vi "CaseSelect.vi"(10 "SelList[]":refnum<vi>[](array[refnum]), 11 "Active VI Ref":refnum<vi>) -> ()   [LabVIEW 2013]
uses:
  Controls/btn-back-36x36.ctl
  Controls/btn-forward-36x36.ctl
  Controls/btn-clear-history-36x36.ctl
  Controls/btn-refresh-36x36.ctl
  <vilib>/Utility/miscctls.llb/LVRectTypeDef.ctl
  StructureTypes.ctl
  JKI State Machine API/source/JKI SM/JKI SM.lvclass
  <vilib>/Utility/traverseref.llb/TRef TravTarget.ctl
  <userlib>/_OpenG.lib/comparison/comparison.llb/String Changed__ogtk.vi
  <userlib>/_OpenG.lib/comparison/comparison.llb/1D String Array Changed__ogtk.vi
  <userlib>/_OpenG.lib/file/file.llb/Build Path - File Names Array - path__ogtk.vi
  <vilib>/regexp/Match Regular Expression.xnode
  <userlib>/_OpenG.lib/string/string.llb/Trim Whitespace (String Array)__ogtk.vi
panel:
  in  "Refresh":T1
  in  "Clear History":T2
  in  "Forward":T3
  in  "Back":T4
  in  "Search Icon":bool
  in  "Clear Search":bool
  in  "Search":string
  in  "Add macro":bool
  in  "Cases":string(tree)
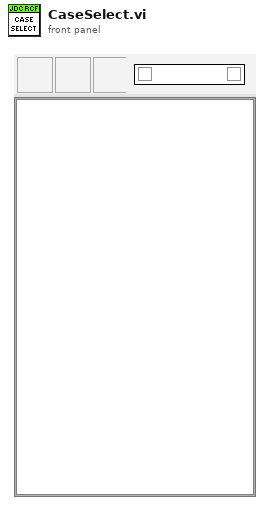
[diagram p1: front panel]
types:
  T1 = typedef "btn-refresh-36x36.ctl" = bool
  T2 = typedef "btn-clear-history-36x36.ctl" = bool
  T3 = typedef "btn-forward-36x36.ctl" = bool
  T4 = typedef "btn-back-36x36.ctl" = bool
  T5 = enum32{"Invalid", "Standard", "Closed", "Hidden", "Minimized", "Maximized"}
  T6 = enum32{"invalid app kind", "Development System", "Run Time System", "Student Edition", "Embedded LabVIEW", "Evaluation", "Custom"}
  T7 = typedef "StructureTypes.ctl" = enum16{"CaseStructure", "EventStructure"}
  T8 = typedef "TRef TravTarget.ctl" = enum16{"FP", "BD", "Other"}
  T9 = typedef "LVPoint32TypeDef.ctl" = cluster{"Horizontal":i32, "Vertical":i32}
  T10 = typedef "LVNodeAndColumnTypeDef.ctl" = cluster{"Node":string, "Column":i32}
  T11 = typedef "LVRectTypeDef.ctl" = cluster{"Left":i16, "Top":i16, "Right":i16, "Bottom":i16}
  T12 = cluster{"Core":cluster{"Current VI Reference":refnum<vi>, "Close Panel on Exit?":bool}, "Indent?":bool, "InBounds":bool, "Activating":bool, "FrameNames":string[], "tag":string, "Top Row Tag":string, "TreeSectHdrs":string, "SectHdr":string, "CaseStrVIName":string, "TempString":string, "DisplayedItems":i32, "SelectedCase":u32, "Display:Primary Workspace":T11, "Cases":refnum<vi>, "StructRef":refnum<vi>, "CaseStrVI Ref":refnum<vi>, "Ctrl?":bool, "NavHist":refnum<vi>[], "NavIndex":i32, "Structure Type":T7, "Undo Transaction":bool, "Top Row Index":i32}
  T13 = cluster{"Current VI Reference":refnum<vi>, "Close Panel on Exit?":bool}
  T14 = enum8{"Enabled", "Disabled", "Disabled and Grayed Out"}
  T15 = cluster{"StringConstant":refnum<vi>, "Structure":string, "Frame Name":string}[]
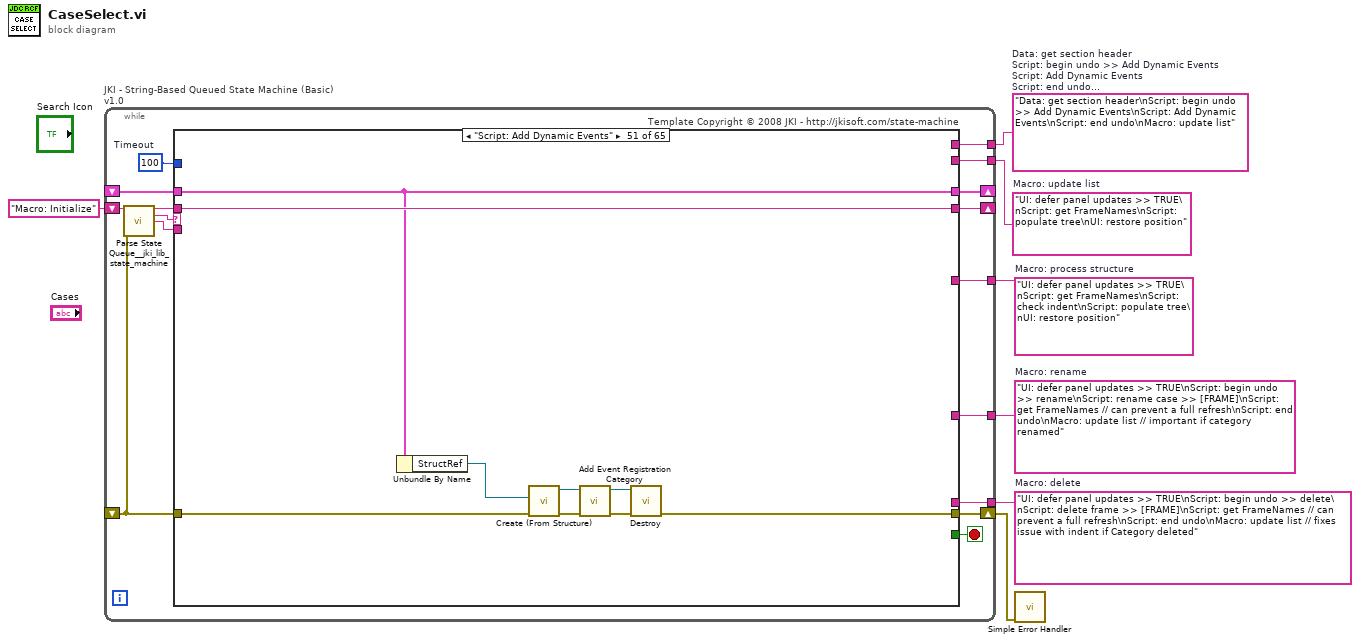
[diagram p0: block diagram]
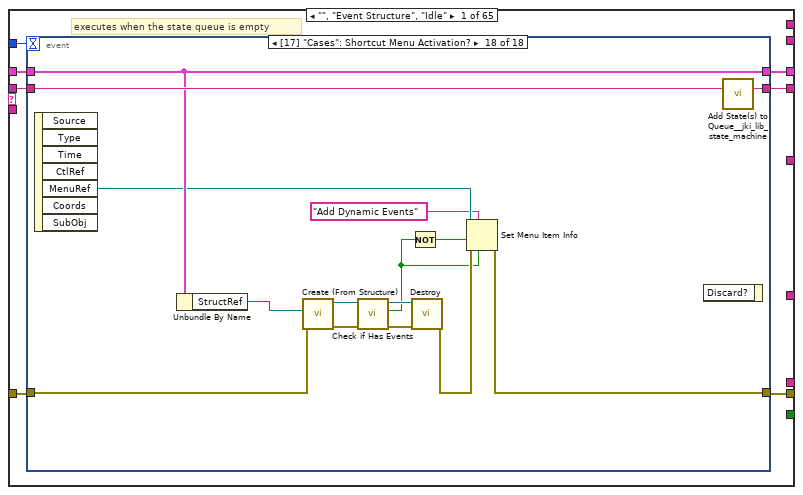
[diagram p2: hidden frame]
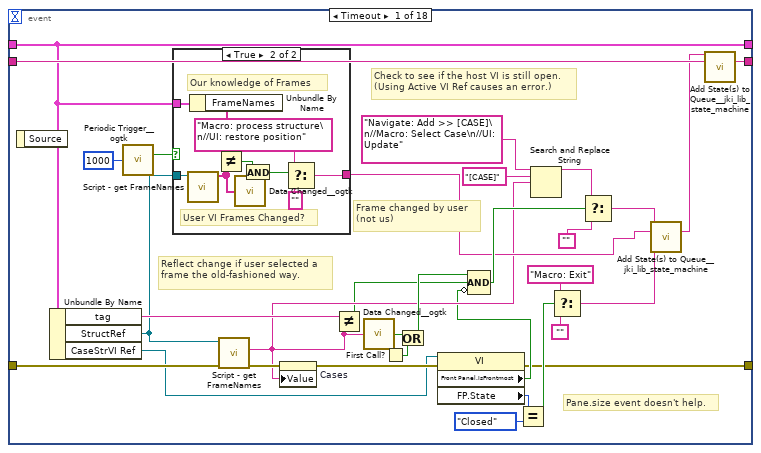
[diagram p3: hidden frame]
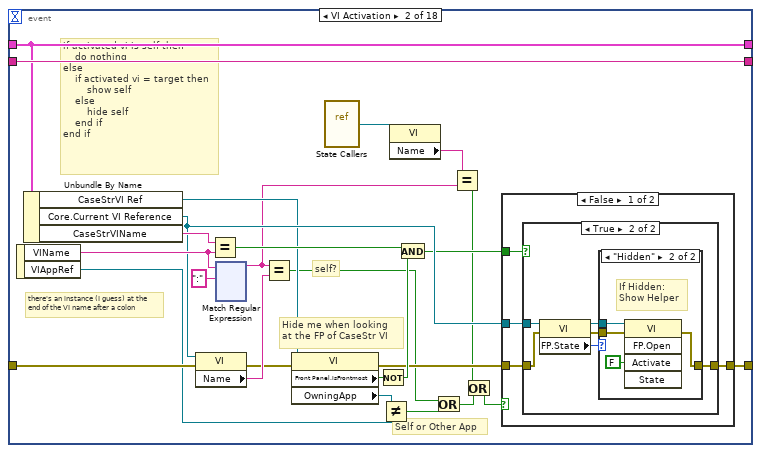
[diagram p5: hidden frame]
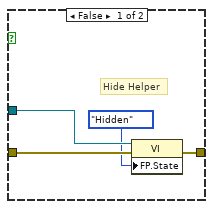
[diagram p6: hidden frame]
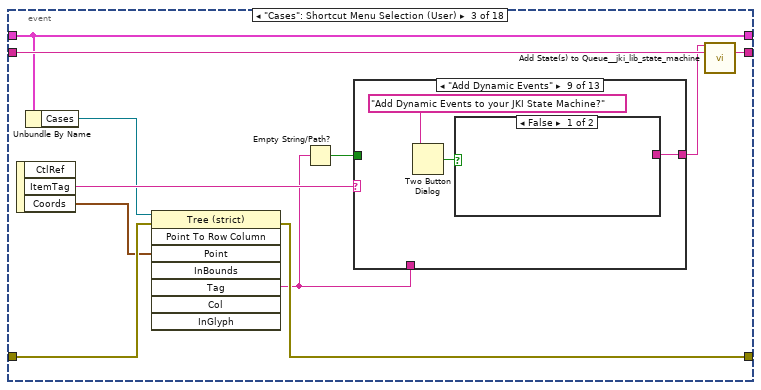
[diagram p9: hidden frame]
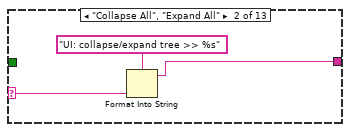
[diagram p11: hidden frame]
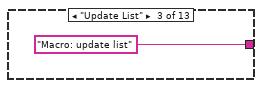
[diagram p12: hidden frame]
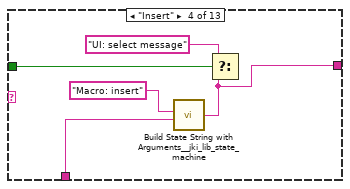
[diagram p13: hidden frame]
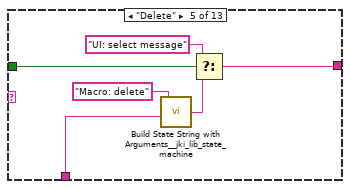
[diagram p14: hidden frame]
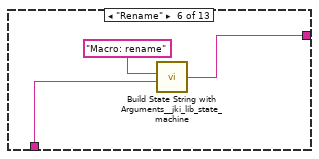
[diagram p15: hidden frame]
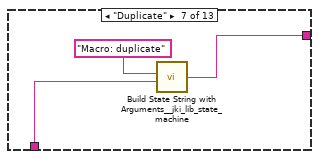
[diagram p16: hidden frame]
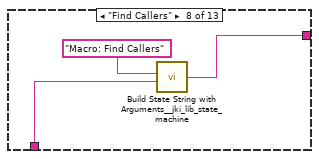
[diagram p17: hidden frame]
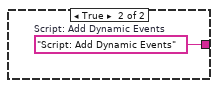
[diagram p18: hidden frame]
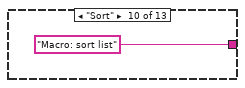
[diagram p19: hidden frame]
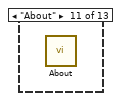
[diagram p20: hidden frame]
diagram:
  w1 = "Data: get section header\nScript: begin undo >> Add Dynamic Events\nScript: Add Dynamic Events\nScript: end undo\nMacro: update list"  # Data: get section header Script: begin undo >> Add Dynamic Events Script: Add Dynamic Events Script: end undo Macro: update list
  w2 = "UI: defer panel updates >> TRUE\nScript: get FrameNames\nScript: populate tree\nUI: restore position"  # Macro: update list
  w4 = "UI: defer panel updates >> TRUE\nScript: begin undo >> delete\nScript: delete frame >> [FRAME]\nScript: get FrameNames // can prevent a full refresh\nScript: end undo\nMacro: update list // fixes issue with indent if Category deleted"  # Macro: delete
  w5 = "UI: defer panel updates >> TRUE\nScript: begin undo >> rename\nScript: rename case >> [FRAME]\nScript: get FrameNames // can prevent a full refresh\nScript: end undo\nMacro: update list // important if category renamed"  # Macro: rename
  w6 = "UI: defer panel updates >> TRUE\nScript: get FrameNames\nScript: check indent\nScript: populate tree\nUI: restore position"  # Macro: process structure
  n1 = while "JKI - String-Based Queued State Machine (Basic) v1.0" {
    shift-right: [w16] -> _
    shift-left: _ -> [w15]
    shift-right: [w19] -> w3
    shift-left: _ -> [w13]
    shift-right: [w18] -> _
    shift-left: "Macro: Initialize" -> [w20]
    tunnel: w6 -> [w12]
    tunnel: w5 -> [w11]
    tunnel: w4 -> [w10]
    tunnel: w2 -> [w9]
    tunnel: w1 -> [w8]
    stop <- w17 stop-if-true
    w14 = 100  # Timeout
    # "Template Copyright © 2008 JKI - http://jkisoft.com/state-machine"
    n2 = call <vilib>:"Parse State Queue__jki_lib_state_machine.vi"("State Queue"=w20, "Error In (no error)"=w13) -> ("Remaining States"=w22:string, "Current State"=w23:string, "Arguments"=w21:string)  [unwired: 1 in, 10 out]
    n3 = case shown="\"Script: Add Dynamic Events\"" w23 {
      selector: w23 -> [_ _ w509 _ _ _ _ _ _ _ _ _ _ _ _ _ _ _ _ _ _ _ _ _ _ _ _ _ _ _ _ _ _ _ _ _ _ _ _ _ _ _ _ _ _ _ _ _ _ _ _ _ _ _ _ _ _ _ _ _ _ _ _ _ _]
      tunnel: w22 -> [w30 w505 w508 w518 w537 _ w560 w564 w574 w618 w635 w644 w647 w655 w672 w674 w716 w726 w744 w759 w787 w810 w812 w819 w822 w830 w840 w861 w864 w870 w874 w885 w893 w898 w907 w911 w916 w926 w933 w934 w947 w964 w965 w975 w998 w1015 w1017 w1041 w1081 w1099 w1108 w1117 w1184 w1244 w1316 w1393 w1430 w1456 w1489 w1513 w1521 w1527 w1535 w1550 w1600]
      tunnel: w21 -> [_ _ _ _ _ _ _ _ _ _ _ _ _ _ _ w673 _ w729 _ w761 _ _ _ _ _ w825 w836 w857 _ _ _ w878 w890 _ w904 _ _ w923 _ _ w937 _ _ w972 _ _ _ _ _ _ _ w1110 w1176 w1234 w1307 w1387 w1423 _ w1493 _ _ _ _ _ _]
      tunnel: w15 -> [w28 w506 w511 w521 w538 w548 w563 w565 _ w617 w633 w645 w648 w656 w670 w676 w715 w731 w748 w762 w786 w809 w813 w816 w823 w831 w841 w853 w865 w868 w876 w879 w894 w899 w908 w913 w918 w928 w930 w935 w945 w961 w966 w973 w997 w1013 w1025 w1040 w1080 w1098 w1107 w1119 w1188 w1236 w1319 w1396 w1431 w1468 w1495 w1514 w1520 w1526 w1534 w1560 w1599]
      tunnel: [w27 w507 w513 w527 w539 w550 w562 w566 w575 w619 w634 w642 w649 w654 w671 w677 w713 w732 w749 w764 w785 w811 w814 w817 w824 w832 w834 w856 w866 w871 w875 w881 w888 w896 w902 w912 w917 w927 w931 w936 w942 w957 w967 w974 w991 w1008 w1018 w1042 w1079 w1097 w1100 w1113 w1187 w1245 w1317 w1394 w1420 w1460 w1479 w1512 w1517 w1523 w1531 w1553 w1594] -> w19
      tunnel: w13 -> [w26 w507 w512 w527 w539 w554 w562 w566 w589 w619 w634 w643 w649 w654 w671 w678 w714 w733 w750 w763 w788 w811 w814 w817 w824 w832 w835 w844 w866 w871 w875 w882 w889 w896 w903 w912 w917 w927 w931 w936 w943 w958 w967 w971 w993 w1016 w1019 w1043 w1073 w1096 w1101 w1120 w1189 w1242 w1312 w1389 w1421 w1466 w1478 w1512 w1519 w1525 w1533 w1559 w1596]
      tunnel: [w29 w505 w508 w518 w537 w546 w560 w564 w574 w618 w635 w644 w647 w655 w672 w674 w716 w725 w743 w758 w787 w810 w812 w818 w821 w829 w839 w860 w863 w869 w873 w884 w892 w897 w906 w910 w915 w925 w932 w934 w947 w964 w965 w975 w998 w1014 w1017 w1041 w1081 w1099 w1108 w1116 w1183 w1244 w1315 w1392 w1429 w1455 w1488 w1513 w1521 w1527 w1535 w1549 w1600] -> w18
      tunnel: [_ _ _ _ _ _ TRUE _ _ _ _ _ _ _ _ _ _ _ _ _ _ _ _ _ _ _ _ _ _ _ _ _ _ _ _ _ _ _ _ _ _ _ _ _ _ _ _ _ _ _ _ _ _ _ _ _ _ _ _ _ _ _ _ _ _] -> w17
      tunnel: [w25 w506 w511 w528 w538 w548 w563 w565 w599 w616 w629 w645 w648 w656 w670 w676 w715 w731 w745 w762 w786 w809 w813 w816 w823 w831 w841 w853 w865 w868 w876 w879 w894 w899 w908 w913 w918 w928 w930 w935 w946 w960 w966 w969 w995 w1011 w1024 w1039 w1076 w1098 w1107 w1119 w1188 w1235 w1319 w1396 w1431 w1454 w1483 w1514 w1516 w1526 w1530 w1560 w1599] -> w16
      tunnel: w14 -> [w24 _ _ _ _ _ _ _ _ _ _ _ _ _ _ _ _ _ _ _ _ _ _ _ _ _ _ _ _ _ _ _ _ _ _ _ _ _ _ _ _ _ _ _ _ _ _ _ _ _ _ _ _ _ _ _ _ _ _ _ _ _ _ _ _]
      tunnel: w12 -> [_ _ _ _ _ _ _ _ _ _ _ _ _ _ _ _ _ _ _ _ _ _ _ _ w820 _ _ _ _ _ _ _ _ _ _ _ _ _ _ _ _ _ _ _ _ _ _ _ _ _ _ _ _ _ _ _ _ _ _ _ _ _ _ _ _]
      tunnel: w11 -> [_ _ _ _ _ _ _ _ _ _ _ _ _ _ _ _ _ _ _ _ _ _ _ _ _ _ _ _ _ _ _ w877 _ _ _ _ _ _ _ _ _ _ _ _ _ _ _ _ _ _ _ _ _ _ _ _ _ _ _ _ _ _ _ _ _]
      tunnel: w10 -> [_ _ _ _ _ _ _ _ _ _ _ _ _ _ _ _ _ _ _ _ _ _ _ _ _ _ w833 _ _ _ _ _ _ _ _ _ _ _ _ _ _ _ _ _ _ _ _ _ _ _ _ _ _ _ _ _ _ _ _ _ _ _ _ _ _]
      tunnel: w9 -> [_ _ _ _ _ _ _ _ _ _ _ _ _ _ _ _ _ _ _ _ _ _ _ _ _ _ _ _ w862 _ _ _ _ _ _ _ _ _ _ _ _ _ _ _ _ _ _ _ _ _ _ _ _ _ _ _ _ _ _ _ _ _ _ _ _]
      tunnel: w8 -> [_ _ _ _ _ _ _ _ _ _ _ _ _ _ _ _ _ _ _ _ _ _ _ _ _ _ _ _ _ _ _ _ _ w895 _ _ _ _ _ _ _ _ _ _ _ _ _ _ _ _ _ _ _ _ _ _ _ _ _ _ _ _ _ _ _]
      frame "", "Event Structure", "Idle" {
        # "executes when the state queue is empty"
        n4 = event shown="[17] \"Cases\": Shortcut Menu Activation?" {
          selector: _ -> [_ _ _ _ _ _ _ _ _ _ _ _ _ _ _ _ _ _]
          dyn-events: _ -> [_ _ _ _ _ _ _ _ _ _ _ _ _ _ _ _ _ _]
          timeout: w24 -> [_ _ _ _ _ _ _ _ _ _ _ _ _ _ _ _ _ _]
          tunnel: w30 -> [w62 w98 w238 w294 w323 w332 w338 w366 w401 w403 w411 w419 w434 w453 w456 w463 w489 w504]
          tunnel: [w61 w98 w237 w293 w322 w332 w337 w365 w401 w402 w410 w418 w433 w452 w457 w463 w488 w503] -> w29
          tunnel: w28 -> [w31 w96 w235 w296 w324 w331 w335 w367 w399 w406 w414 w422 w447 w450 w458 w464 w486 w497]
          tunnel: [w32 w94 w231 w283 w320 w327 w339 w368 w400 w405 w413 w421 w435 w454 w459 w460 w487 w492] -> w27
          tunnel: w26 -> [w60 w86 w240 w298 w320 w328 w340 w368 w400 w405 w413 w421 w426 w454 w459 w461 w487 w496]
          tunnel: [w31 w96 w235 w287 w321 w326 w335 w363 w399 w406 w414 w422 w448 w450 w458 w462 w486 w497] -> w25
          event Timeout {
            # "Frame changed by user\n(not us)"
            # "Reflect change if user selected a frame the old-fashioned way."
            # "Pane.size event doesn't help."
            # "Check to see if the host VI is still open.\n(Using Active VI Ref causes an error.)"
            n5 = event-data() -> ()  [unwired: 2 out]
            n6 = Unbundle By Name(w31) -> ("tag"=w53:string, "StructRef"=w39:refnum<vi>, "CaseStrVI Ref"=w40:refnum<vi>)
            n7 = call <userlib>:"Periodic Trigger__ogtk.vi"("time (ms)"=u32 1000) -> ("Triggered"=w42:bool)  [unwired: 12 in, 2 out]
            n8 = case shown="True" w42 {
              tunnel: w39 -> [_ w72]
              tunnel: [_ w69] -> w41
              tunnel: w31 -> [_ w68]
              frame False {
              }
              frame True {
                # "Our knowledge of Frames"
                # "User VI Frames Changed?"
                n9 = call "Script - get FrameNames.vi"("StructRef"=w72) -> ("Frame Names"=w67:string[])  [unwired: 5 in, 5 out]
                n10 = Unbundle By Name(w68) -> ("FrameNames"=w66:string[])
                n11 = Not Equal?(x=w66, y=w67) -> (x != y?=w64:bool)
                n12 = call-poly <userlib>:"Data Changed__ogtk.vi"("1D String Array"=w67) -> ("Changed"=w63:bool)
                n13 = And(x=w64, y=w63) -> (x .and. y?=w65:bool)
                n14 = Select(t="Macro: process structure\n//UI: restore position", s=w65, f="") -> (s? t:f=w69:string)
              }
            }
            n15 = call "Script - get FrameNames.vi"("error in"=w60, "StructRef"=w39) -> ("error out"=w38:errorcluster, "Visible Frame Name"=w37:string)  [unwired: 4 in, 4 out]
            n16 = property on="Cases" class="Tree (strict)"(error in=w38, "Value"=w37) -> (error out=w54:errorcluster)  [unwired: 1 in, 1 out]
            n17 = Not Equal?(x=w53, y=w37) -> (x != y?=w33:bool)
            n18 = call-poly <userlib>:"Data Changed__ogtk.vi"("String"=w37) -> ("Changed"=w45:bool)
            n19 = First Call?() -> (First Call?: T/F=w46:bool)
            n20 = Or(x=w45, y=w46) -> (x .or. y?=w44:bool)
            n21 = property class="VI"(reference=w40, error in=w54) -> (error out=w32:errorcluster, "Front Panel.IsFrontmost"=w34:bool, "FP.State"=w59:T5)  [unwired: 1 out]
            n22 = Compound Arithmetic op=AND(w44, w33, invert w34) -> (w49:bool)
            n23 = Equal?(x=w59, y=T5."Closed" ("Front Panel Window:State")) -> (x = y?=w57:bool)
            n24 = Search and Replace String(input string="Navigate: Add >> [CASE]\n//Macro: Select Case\n//UI: Update" ("State(s) in Front (\"\")"), search string="[CASE]", replace string=w37) -> (result string=w36:string)  [unwired: 5 in, 3 out]
            n25 = Select(t="Macro: Exit", s=w57, f="") -> (s? t:f=w48:string)
            n26 = Select(t=w36, s=w49, f="") -> (s? t:f=w35:string)
            n27 = call <vilib>:"Add State(s) to Queue__jki_lib_state_machine.vi"("State(s) in Front (\"\")"=w35, "State(s) in (\"\")"=w41, "State(s) at Back (\"\")"=w48) -> ("States Out"=w47:string)  [unwired: 12 out]
            n28 = call <vilib>:"Add State(s) to Queue__jki_lib_state_machine.vi"("State(s) in Front (\"\")"=w47, "State(s) in (\"\")"=w62) -> ("States Out"=w61:string)  [unwired: 1 in, 12 out]
          }
          event VI Activation {
            # "Self or Other App"
            # "self?"
            # "Hide me when looking\nat the FP of CaseStr VI"
            # "there's an instance (I guess) at the\nend of the VI name after a colon"
            # "if activated vi is self then\n    do nothing\nelse\n    if activated vi = target then\n        show self\n    else\n        hide self\n    end if\nend if"
            n29 = event-data() -> ("VIName"=w91:string, "VIAppRef"=w81:refnum<vi>)  [unwired: 1 out]
            n30 = Unbundle By Name(w96) -> ("CaseStrVI Ref"=w84:refnum<vi>, "Core.Current VI Reference"=w90:refnum<vi>, "CaseStrVIName"=w97:string)
            n31 = property class="VI"(reference=w90, error in=w86) -> (error out=w85:errorcluster, "Name"=w92:string)  [unwired: 1 out]
            n32 = Equal?(x=w97, y=w91) -> (x = y?=w95:bool)
            n33 = xnode "Match Regular Expression"("input string"=w91, "regular expression"=":") -> ("before match"=w76:string)  [unwired: 3 in, 5 out]
            n34 = Equal?(x=w76, y=w92) -> (x = y?=w79:bool)
            n35 = property class="VI"(reference=w84, error in=w85) -> (error out=w87:errorcluster, "Front Panel.IsFrontmost"=w89:bool, "OwningApp"=w82:refnum<vi>)  [unwired: 1 out]
            n36 = vi-ref "State Callers.vi"() -> (w78:refnum<vi>)
            n37 = Not(x=w89) -> (.not. x?=w88:bool)
            n38 = Not Equal?(x=w82, y=w81) -> (x != y?=w80:bool)
            n39 = property class="VI"(reference=w78) -> ("Name"=w77:string)  [unwired: 1 in, 2 out]
            n40 = And(x=w95, y=w88) -> (x .and. y?=w83:bool)
            n41 = Or(x=w79, y=w80) -> (x .or. y?=w74:bool)
            n42 = Equal?(x=w77, y=w76) -> (x = y?=w75:bool)
            n43 = Or(x=w75, y=w74) -> (x .or. y?=w73:bool)
            n44 = case shown="False" w73 {
              tunnel: w87 -> [w102 w118]
              tunnel: [w100 w118] -> w94
              tunnel: w90 -> [w101 _]
              tunnel: w83 -> [w99 _]
              frame False {
                n45 = case shown="True" w99 {
                  tunnel: w102 -> [w106 w111]
                  tunnel: w101 -> [w105 w112]
                  tunnel: [w104 w109] -> w100
                  frame False {
                    # "Hide Helper"
                    n46 = property class="VI"(reference=w105, error in=w106, "FP.State"=T5."Hidden" ("Front Panel Window:State")) -> (error out=w104:errorcluster)  [unwired: 1 out]
                  }
                  frame True {
                    n47 = property class="VI"(reference=w112, error in=w111) -> (reference out=w108:refnum<vi>, error out=w107:errorcluster, "FP.State"=w110:T5)
                    n48 = case shown="\"Hidden\"" w110 {
                      tunnel: [w113 w117] -> w109
                      tunnel: w108 -> [_ w116]
                      tunnel: w107 -> [w113 w115]
                      frame Default {
                      }
                      frame "Hidden" {
                        # "If Hidden:\nShow Helper"
                        n49 = invoke class="VI" method="FP.Open"(reference=w116, error in=w115, "Activate"=FALSE ("Activate?")) -> (error out=w117:errorcluster)  [unwired: 2 in, 4 out]
                      }
                    }
                  }
                }
              }
              frame True {
              }
            }
          }
          event "Cases": Shortcut Menu Selection (User) {
            n50 = event-data() -> ("ItemTag"=w239:string, "Coords"=w232:T9)  [unwired: 2 out]
            n51 = Unbundle By Name(w235) -> ("Cases"=w234:refnum<vi>)
            n52 = invoke class="Tree (strict)" method="Point To Row Column"(reference=w234, error in=w240, "Point"=w232) -> (error out=w231:errorcluster, "Tag"=w230:string)  [unwired: 5 in, 6 out]
            n53 = Empty String/Path?(string/path=w230) -> (empty?=w233:bool)
            n54 = case shown="\"Add Dynamic Events\"" w239 {
              selector: w239 -> [_ w242 _ _ _ _ _ _ _ _ _ _ _]
              tunnel: [_ w241 "Macro: update list" w245 w253 w256 w259 w262 w267 "Macro: sort list" _ w270 _] -> w236
              tunnel: w233 -> [_ _ _ w249 w255 _ _ _ _ _ _ _ _]
              tunnel: w230 -> [_ _ _ w246 w251 w258 w261 w264 _ _ _ _ w276]
              frame Default {
              }
              frame "Collapse All", "Expand All" {
                n55 = Format Into String(format string="UI: collapse/expand tree >> %s", w242) -> (resulting string=w241:string)  [unwired: 2 in, 1 out]
              }
              frame "Update List" {
              }
              frame "Insert" {
                n56 = call <vilib>:"Build State String with Arguments__jki_lib_state_machine.vi"("Arguments (\"\")"=w246, "State"="Macro: insert") -> ("State with Arguments"=w245:string)  [unwired: 4 in]
                n57 = Select(t="UI: select message", s=w249, f=w245) -> ()  [unwired: 1 out]
              }
              frame "Delete" {
                n58 = call <vilib>:"Build State String with Arguments__jki_lib_state_machine.vi"("Arguments (\"\")"=w251, "State"="Macro: delete") -> ("State with Arguments"=w250:string)  [unwired: 4 in]
                n59 = Select(t="UI: select message", s=w255, f=w250) -> (s? t:f=w253:string)
              }
              frame "Rename" {
                n60 = call <vilib>:"Build State String with Arguments__jki_lib_state_machine.vi"("Arguments (\"\")"=w258, "State"="Macro: rename") -> ("State with Arguments"=w256:string)  [unwired: 4 in]
              }
              frame "Duplicate" {
                n61 = call <vilib>:"Build State String with Arguments__jki_lib_state_machine.vi"("Arguments (\"\")"=w261, "State"="Macro: duplicate") -> ("State with Arguments"=w259:string)  [unwired: 4 in]
              }
              frame "Find Callers" {
                n62 = call <vilib>:"Build State String with Arguments__jki_lib_state_machine.vi"("Arguments (\"\")"=w264, "State"="Macro: Find Callers") -> ("State with Arguments"=w262:string)  [unwired: 4 in]
              }
              frame "Add Dynamic Events" {
                n63 = Two Button Dialog(message="Add Dynamic Events to your JKI State Machine?" ("format string")) -> (T button?=w266:bool)  [unwired: 2 in]
                n64 = case shown="False" w266 {
                  tunnel: [_ w268] -> w267
                  frame False {
                  }
                  frame True {
                    w268 = "Script: Add Dynamic Events"  # Script: Add Dynamic Events
                  }
                }
              }
              frame "Sort" {
              }
              frame "About" {
                n65 = call "About.vi"() -> ()  [unwired: 1 out]
              }
              frame "highlight" {
                w270 = "Script: highlight"  # Script: highlight
              }
              frame "Copy State Name to Clipboard" {
                # "Don't trim quotes"
                n66 = call <vilib>:"Trim Whitespace.vi"("string"=w276) -> ("trimmed string"=w273:string)  [unwired: 1 in]
                n67 = Equal?(x=string[] ["\"\", \"Idle\"", " \"\", \"Event Structure\", \"Idle\" "], y=w273) -> (x = y?=w275:bool[])
                n68 = call "Remove Quotes from String if Present.vi"("String"=w273) -> ("String with Quotes Removed"=w272:string)  [unwired: 10 in]
                n69 = Or Array Elements(Boolean array=w275) -> (logical OR=w274:bool)
                n70 = Select(t=w273, s=w274, f=w272) -> (s? t:f=w271:string)
                n71 = invoke class="App" method="Clipboard.Write"("Param 0"=w271) -> ()  [unwired: 3 in, 4 out]
              }
            }
            n72 = call <vilib>:"Add State(s) to Queue__jki_lib_state_machine.vi"("State(s) in Front (\"\")"=w236, "State(s) in (\"\")"=w238) -> ("States Out"=w237:string)  [unwired: 1 in, 12 out]
          }
          event "Cases": Drag Ended {
            n73 = event-data() -> ("CtlRef"=w297:refnum<vi>)  [unwired: 1 out]
            n74 = Unbundle By Name(w296) -> ("Ctrl?"=w280:bool, "FrameNames"=w291:string[], "StructRef"=w295:refnum<vi>, "CaseStrVI Ref"=w279:refnum<vi>)
            n75 = property class="Tree (strict)"(reference=w297, error in=w298) -> (error out=w292:errorcluster, "TopLeft"=w286:T10, "Value"=w282:string, "All Tags"=w284:string[])  [unwired: 1 out]
            n76 = Unbundle By Name(w286) -> ("Node"=w285:string)
            n77 = Array Size(array=w291) -> (size(s)=w289:i32)
            n78 = Array Size(array=w284) -> (size(s)=w290:i32)
            n79 = Bundle By Name(cluster=w296, "Top Row Tag"=w285, "tag"=w282) -> (w287:T12)
            n80 = Equal?(x=w289, y=w290) -> (x = y?=w288:bool)
            n81 = case shown="True" w288 {
              tunnel: w295 -> [_ w302]
              tunnel: w292 -> [w300 w309]
              tunnel: [w300 w305] -> w283
              tunnel: w291 -> [_ w311]
              tunnel: w284 -> [_ w310]
              tunnel: ["Macro: process drag-copy" ("message") "Macro: update list\nMacro: Select Case" ("message")] -> w278
              tunnel: w279 -> [_ w301]
              frame False {
                # "There are more tags in the tree than\nthere are frames in the Case Structure.\nA drag/copy operation just occurred."
              }
              frame True {
                n82 = for {
                  tunnel: w311 -> [w315]
                  tunnel: w310 -> [w314] mode=indexing
                  tunnel: [w313] -> w312 mode=indexing
                  n83 = Search 1D Array(1D array=w315, element=w314) -> (index of element=w313:i32)  [unwired: 1 out]
                }
                n84 = invoke class="VI" method="Transaction.Begin Undo"(reference=w301, error in=w309, "Name"="Drag") -> (reference out=w306:refnum<vi>, error out=w307:errorcluster)  [unwired: 1 in, 2 out]
                n85 = invoke class="MFStruct" method="RearrangeFramesByIdx"(reference=w302, error in=w307, "Index Array"=w312) -> (error out=w303:errorcluster)  [unwired: 1 in, 3 out]
                n86 = invoke class="VI" method="Transaction.End Undo"(reference=w306, error in=w303) -> (error out=w305:errorcluster)  [unwired: 1 in, 2 out]
              }
            }
            n87 = Select(t="Macro: drop state name", s=w280, f=w278) -> ()  [unwired: 1 out]
            n88 = call <vilib>:"Add State(s) to Queue__jki_lib_state_machine.vi"("State(s) in Front (\"\")"=w278, "State(s) in (\"\")"=w294) -> ("States Out"=w293:string)  [unwired: 1 in, 12 out]
          }
          event "Cases": Value Change {
            n89 = event-data() -> ("NewVal"=w317:string)  [unwired: 1 out]
            n90 = Bundle By Name(cluster=w324, "tag"=w317) -> (w321:T12)
            n91 = Search and Replace String(input string="Navigate: Add >> [CASE]\nMacro: Select Case\nUI: Update" ("State(s) in Front (\"\")"), search string="[CASE]", replace string=w317) -> (result string=w316:string)  [unwired: 5 in, 3 out]
            n92 = call <vilib>:"Add State(s) to Queue__jki_lib_state_machine.vi"("State(s) in Front (\"\")"=w316, "State(s) in (\"\")"=w323) -> ("States Out"=w322:string)  [unwired: 1 in, 12 out]
          }
          event "Cases": Mouse Down {
            # "This makes a mouse click work\nonly if the click was in bounds."
            n93 = event-data() -> ("CtlRef"=w330:refnum<vi>, "Coords"=w329:T9)  [unwired: 4 out]
            n94 = invoke class="Tree (strict)" method="Point To Row Column"(reference=w330, error in=w328, "Point"=w329) -> (error out=w327:errorcluster, "InBounds"=w325:bool)  [unwired: 5 in, 6 out]
            n95 = Bundle By Name(cluster=w331, "InBounds"=w325) -> (w326:T12)
          }
          event "Cases": Mouse Up {
            n96 = event-data() -> ("Mods.Double Click"=w333:bool, "PlatMods.Ctrl"=w334:bool, "CtlRef"=w342:refnum<vi>, "Coords"=w341:T9)  [unwired: 1 out]
            n97 = case shown="False" w333 {
              tunnel: w342 -> [w354 _]
              tunnel: w341 -> [w353 _]
              tunnel: w340 -> [w352 w356]
              tunnel: [w351 w356] -> w339
              tunnel: [w350 "//Macro: append string"] -> w336
              tunnel: w335 -> [w349 _]
              tunnel: w334 -> [w348 _]
              frame False {
                n98 = invoke class="Tree (strict)" method="Point To Row Column"(reference=w354, error in=w352, "Point"=w353) -> (error out=w351:errorcluster, "InBounds"=w346:bool)  [unwired: 5 in, 6 out]
                n99 = Unbundle By Name(w349) -> ("InBounds"=w347:bool)
                n100 = Compound Arithmetic op=AND(invert w348, w347, w346) -> (w345:bool)
                n101 = Select(t="//Macro: Select Case", s=w345, f="") -> (s? t:f=w350:string)
              }
              frame True {
              }
            }
            n102 = call <vilib>:"Add State(s) to Queue__jki_lib_state_machine.vi"("State(s) in Front (\"\")"=w336, "State(s) in (\"\")"=w338) -> ("States Out"=w337:string)  [unwired: 1 in, 12 out]
          }
          event Key Down? {
            n103 = event-data() -> ("PlatMods.Shift"=w359:bool, "PlatMods.Ctrl"=w361:bool, "ScanCode"=w360:i16)  [unwired: 1 out]
            n104 = Bundle By Name(cluster=w367, "Ctrl?"=w361) -> (w363:T12)
            n105 = Unbundle By Name(w363) -> ("tag"=w362:string, "CaseStrVI Ref"=w358:refnum<vi>)
            n106 = case shown="44" w360 {
              tunnel: [_ w370 w374 w378 w383 _] -> w364
              tunnel: w362 -> [_ w372 w376 w380 w384 w393]
              tunnel: w361 -> [_ _ _ _ w382 w392]
              tunnel: w359 -> [_ _ _ _ _ w391]
              tunnel: w358 -> [_ _ _ _ _ w390]
              tunnel: [_ TRUE TRUE TRUE w381 w389] -> w357
              frame 0, Default {
              }
              frame 60 {
                # "F2"
                n107 = call <vilib>:"Build State String with Arguments__jki_lib_state_machine.vi"("Arguments (\"\")"=w372, "State"="Macro: rename") -> ("State with Arguments"=w370:string)  [unwired: 4 in]
              }
              frame 82 {
                n108 = call <vilib>:"Build State String with Arguments__jki_lib_state_machine.vi"("Arguments (\"\")"=w376, "State"="Macro: insert") -> ("State with Arguments"=w374:string)  [unwired: 4 in]
              }
              frame 83 {
                # "Delete"
                n109 = call <vilib>:"Build State String with Arguments__jki_lib_state_machine.vi"("Arguments (\"\")"=w380, "State"="Macro: delete") -> ("State with Arguments"=w378:string)  [unwired: 4 in]
              }
              frame 33 {
                # "Ctrl+F"
                n110 = case shown="True" w382 {
                  tunnel: w384 -> [_ w388]
                  tunnel: [_ w386] -> w383
                  tunnel: [_ TRUE] -> w381
                  frame False {
                  }
                  frame True {
                    n111 = call <vilib>:"Build State String with Arguments__jki_lib_state_machine.vi"("Arguments (\"\")"=w388, "State"="Macro: Find Callers") -> ("State with Arguments"=w386:string)  [unwired: 4 in]
                  }
                }
              }
              frame 44 {
                # "Z"
                n112 = case shown="True" w392 {
                  tunnel: w393 -> [_ _]
                  tunnel: w391 -> [_ w396]
                  tunnel: w390 -> [_ w395]
                  tunnel: [_ TRUE] -> w389
                  frame False {
                  }
                  frame True {
                    # "Ctrl+Z"
                    n113 = case shown="True" w396 {
                      tunnel: w395 -> [w397 w398]
                      frame False {
                        n114 = invoke class="VI" method="Transaction.Undo"(reference=w397) -> ()  [unwired: 2 in, 3 out]
                      }
                      frame True {
                        n115 = invoke class="VI" method="Transaction.Redo"(reference=w398) -> ()  [unwired: 2 in, 3 out]
                      }
                    }
                  }
                }
              }
            }
            n116 = event-data("Discard?"=w357) -> ()  [unwired: 1 in, 1 out]
            n117 = call <vilib>:"Add State(s) to Queue__jki_lib_state_machine.vi"("State(s) in Front (\"\")"=w364, "State(s) in (\"\")"=w366) -> ("States Out"=w365:string)  [unwired: 1 in, 12 out]
          }
          event Mouse Leave {
            n118 = event-data() -> ()  [unwired: 5 out]
          }
          event Panel Resize {
            n119 = event-data() -> ()  [unwired: 4 out]
            n120 = call <vilib>:"Add State(s) to Queue__jki_lib_state_machine.vi"("State(s) in Front (\"\")"="UI: show/hide scroll bar", "State(s) in (\"\")"=w403) -> ("States Out"=w402:string)  [unwired: 1 in, 12 out]
          }
          event "Search": Value Change {
            n121 = event-data() -> ("NewVal"=w409:string)  [unwired: 6 out]
            n122 = Empty String/Path?(string/path=w409) -> (empty?=w407:bool)
            n123 = Not(x=w407) -> (.not. x?=w408:bool)
            n124 = property on="Search Icon" class="Bool (strict)"("Visible"=w407) -> ()  [unwired: 2 in, 2 out]
            n125 = property on="Clear Search" class="Bool (strict)"("Visible"=w408) -> ()  [unwired: 2 in, 2 out]
            n126 = call <vilib>:"Add State(s) to Queue__jki_lib_state_machine.vi"("State(s) in Front (\"\")"="Macro: process structure", "State(s) in (\"\")"=w411) -> ("States Out"=w410:string)  [unwired: 1 in, 12 out]
          }
          event "Clear Search": Value Change {
            n127 = event-data() -> ()  [unwired: 7 out]
            n128 = property on="Clear Search" class="Bool (strict)"("Visible"=FALSE) -> ()  [unwired: 2 in, 2 out]
            n129 = property on="Search Icon" class="Bool (strict)"("Visible"=TRUE) -> ()  [unwired: 2 in, 2 out]
            n130 = local write "Search"("" ("Search")) -> ()
            n131 = call <vilib>:"Add State(s) to Queue__jki_lib_state_machine.vi"("State(s) in Front (\"\")"="Macro: process structure", "State(s) in (\"\")"=w419) -> ("States Out"=w418:string)  [unwired: 1 in, 12 out]
          }
          event Value Change {
            n132 = event-data() -> ()  [unwired: 7 out]
            n133 = Unbundle By Name(w447) -> ("NavIndex"=w436:i32, "NavHist"=w438:refnum<vi>[], "StructRef"=w429:refnum<vi>)  [unwired: 1 out]
            n134 = Decrement(x=w436) -> (x-1=w446:i32)
            n135 = Increment(x=w436) -> (x+1=w445:i32)
            n136 = Select(t=w446, s="Back", f=w445) -> (s? t:f=w442:i32)
            n137 = call "Script - get FrameNames.vi"("error in"=w426, "StructRef"=w429) -> ("error out"=w425:errorcluster, "Frame Names"=w424:string[], "Frames[]"=w428:refnum<vi>[])  [unwired: 4 in, 3 out]
            n138 = Array Size(array=w438) -> (size(s)=w444:i32)
            n139 = Decrement(x=w444) -> (x-1=w437:i32)
            n140 = In Range and Coerce(upper limit=w437, x=w442, lower limit=0) -> (coerced(x)=w439:i32, In Range?=w441:bool)
            n141 = Index Array(array=w438, index=w439) -> (element=w430:refnum<vi>)
            n142 = Search 1D Array(1D array=w428, element=w430) -> (index of element=w423:i32)  [unwired: 1 out]
            n143 = Index Array(array=w424, index=w423) -> (element=w427:string)
            n144 = To Unsigned Long Integer(number=w423) -> (unsigned 32bit integer=w449:u32)
            n145 = Not(x=w441) -> (.not. x?=w440:bool)
            n146 = property class="MFStruct"(reference=w429, error in=w425, "VisFrame"=w449) -> (error out=w435:errorcluster)  [unwired: 1 out]
            n147 = call "Display Message to User"("Enable"=w440) -> ()  [unwired: 9 in, 2 out]
            n148 = Bundle By Name(cluster=w447, "NavIndex"=w439, "SelectedCase"=w449, "tag"=w427) -> (w448:T12)
            n149 = call <vilib>:"Add State(s) to Queue__jki_lib_state_machine.vi"("State(s) in Front (\"\")"="UI: Update" ("State(s) in Front (\"\")"), "State(s) in (\"\")"=w434) -> ("States Out"=w433:string)  [unwired: 13 in]
          }
          event Value Change {
            n150 = event-data() -> ()  [unwired: 7 out]
            n151 = call <vilib>:"Add State(s) to Queue__jki_lib_state_machine.vi"("State(s) in Front (\"\")"="Navigation: Clear History\nUI: Update" ("State(s) in Front (\"\")"), "State(s) in (\"\")"=w453) -> ("States Out"=w452:string)  [unwired: 13 in]
          }
          event Value Change {
            n152 = event-data() -> ()  [unwired: 7 out]
            n153 = call <vilib>:"Add State(s) to Queue__jki_lib_state_machine.vi"("State(s) in Front (\"\")"="Macro: update list" ("State(s) in Front (\"\")"), "State(s) in (\"\")"=w456) -> ("States Out"=w457:string)  [unwired: 13 in]
          }
          event "Add macro": Value Change {
            n154 = event-data() -> ()  [unwired: 2 out]
            n155 = disable-structure shown="Enabled" {
              disable-tunnel: w464 -> [w482 w483]
              disable-tunnel: [w481 w483] -> w462
              disable-tunnel: w461 -> [w480 _]
              disable-tunnel: [w479 _] -> w460
              frame Disabled {
                (unwired) 0 ("NavIndex")
                w469 = "\""
                n156 = call "CaseSelect JKI-RCF Plugin"("error in (no error)"=w480) -> ("Macro"=w468:string, "error out"=w479:errorcluster)  [unwired: 16 in, 1 out]
                n157 = Search and Replace String(replace all?=TRUE ("replace all? (F)"), input string=w468, search string="\n", replace string="\"\n\"" ("replace string (\"\")")) -> (result string=w470:string)  [unwired: 4 in, 3 out]
                n158 = Concatenate Strings(w469, w470, w469) -> (w467:string)
                n159 = Spreadsheet String To Array(delimiter (Tab)="\n", format string="%s", spreadsheet string=w467, array type (2D Dbl)=string[] []) -> (array=w476:string[])
                n160 = Array Size(array=w476) -> (size(s)=w474:i32)
                n161 = Reverse 1D Array(array=w476) -> (reversed array=w466:string[])
                n162 = Decrement(x=w474) -> (x-1=w465:i32)
                n163 = Bundle By Name(cluster=w482, "NavHist"=w466, "NavIndex"=w465) -> (w481:T12)
              }
              frame Enabled {
              }
            }
          }
          event Panel Close? {
            # "Discard the event because we'll close the front panel ourselves in Macro: Exit"
            # "Close Panel button (pressed) Event\n(this executes Macro: Exit to terminate the VI)"
            n164 = event-data() -> ()  [unwired: 2 out]
            n165 = event-data("Discard?"=TRUE) -> ()  [unwired: 1 in, 1 out]
            n166 = call <vilib>:"Add State(s) to Queue__jki_lib_state_machine.vi"("State(s) in Front (\"\")"="Macro: Exit", "State(s) in (\"\")"=w489) -> ("States Out"=w488:string)  [unwired: 1 in, 12 out]
          }
          event "Cases": Shortcut Menu Activation? {
            n167 = event-data() -> ("MenuRef"=w494:refnum<k9>)  [unwired: 7 out]
            n168 = Unbundle By Name(w497) -> ("StructRef"=w502:refnum<vi>)
            n169 = call "Create (From Structure).vi"("error in (no error)"=w496, "Structure"=w502) -> ("error out"=w500:errorcluster, "JKI SM out"=w501:refnum<class "JKI SM.lvclass">)  [unwired: 8 in]
            n170 = call "Check if Has Events.vi"("error in (no error)"=w500, "JKI SM in"=w501) -> ("error out"=w498:errorcluster, "Has Dyanamic Events?"=w491:bool, "JKI SM out"=w499:refnum<class "JKI SM.lvclass">)  [unwired: 7 in]
            n171 = Not(x=w491) -> (.not. x?=w495:bool)
            n172 = call "Destroy.vi"("error in (no error)"=w498, "JKI SM in"=w499) -> ("error out"=w493:errorcluster)  [unwired: 9 in]
            n173 = Set Menu Item Info(6:w491, 7:"Add Dynamic Events" ("item name"), 8:w493, 9:w495, 11:w494) -> (0:w492:errorcluster)  [unwired: 2 in, 1 out]
            n174 = event-data() -> ()  [unwired: 2 in, 1 out]
            n175 = call <vilib>:"Add State(s) to Queue__jki_lib_state_machine.vi"("State(s) in (\"\")"=w504) -> ("States Out"=w503:string)  [unwired: 2 in, 12 out]
          }
        }
      }
      frame "---------- Core ----------" {
        # "Do not put any code in this frame.\n(it is a separator no-op)"
      }
      frame Default {
        w516 = 42 items=["No error", "Argument error", "Memory is full", "Out of zone", "End of file", "File already open", "Generic file I/O error", "File not found", "File permission error", "Disk is full", "Duplicate path", "Too many files open", "System feature not enabled", "Resource file not found", "Cannot add resource", "Resource not found", "Image not found", "Image memory error", "Pen does not exist", "Config type invalid", "Config token not found", "Config parse error", "Config memory error", "Bad external code format", "Bad external code offset", "External code not present", "Null window", "Destroy window error", "Null menu", "Print aborted", "Bad print record", "Print driver error", "Windows error during printing", "Memory error during printing", "Print dialog error", "Generic print error", "Invalid device refnum", "Device not found", "Device parameter error", "Device unit error", "Cannot open device", "Device call aborted", "Generic error", "Cancelled by user", "Object ID too low", "Object ID too high", "Object not in heap", "Unknown heap", "Unknown object (invalid DefProc)", "Unknown object (DefProc not in table)", "Message out of range", "Invalid (null) method", "Unknown message", "Manager call not supported", "Bad address", "Network operation in progress", "Network operation timed out", "Connection is busy", "Network attribute not supported", "Network error", "Address in use", "System out of memory", "Connection aborted", "Connection refused", "Not connected", "Already connected", "Connection closed", "Initialization error (interapplication manager)", "Bad occurrence", "Wait on unbound occurrence handler", "Occurrence queue overflow", "Datalog type conflict", "Unused", "Unrecognized type (interapplication manager)", "Memory corrupt", "Failed to make temporary DLL", "Old CIN version", "Drag socket not found", "Failed to load drop-object", "Failed to register OLE object", "Failed to release OLE object", "Format specifier type mismatch", "Unknown format specifier", "Too few format specifiers", "Too many format specifiers", "Scan failed", "Newer CIN version", "Error converting to variant", "Runtime menu error", "Password tampered", "Variant attribute not found", "Incompatible variant data type", "Event data is not available", "Event Store is not present", "Occurrence is not found", "Event Queue is not created", "Event info is not available", "Refnum passed is NULL", "Error retrieving Class GUID", "Error retrieving CoClass GUID", "Error retrieving TypeLib GUID.", "Bad built application magic bytes.", "Specific driver is different from the specific driver associated with the Logical Name.", "There is no session opened to the class driver.", "Max Error", "MAX - Error with config objects", "MAX - Error loading configuration", "MAX - Group not supported"]
        # "Current State"
        # "Do not delete, rename, or modify this frame.\n(this is used to capture unhandled states and typos)"
        # "Handle mistyped state name (developer tool)"
        n176 = Format Into String(format string="Software Exception: Unhandled State \"%s\"." ("message"), error in=w512, w509) -> (resulting string=w515:string, error out=w514:errorcluster)  [unwired: 1 in]
        n177 = call <vilib>:"Error Cluster From Error Code.vi"("show call chain? (False)"=TRUE, "error in (no error)"=w514, "error message (\"\")"=w515, "error code (0)"=w516) -> ("error out"=w513:errorcluster)  [unwired: 5 out]
      }
      frame "Initialize Core Data" {
        # "Do not delete, rename, or modify this frame.\n(this is used to determine panel behavior on exit)"
        # "originally closed?"
        # "exe?"
        # "If panel starts closed or is an EXE, then close it when we exit"
        n178 = property class="VI"() -> ("Front Panel.Open"=w526:bool)  [unwired: 2 in, 2 out]
        n179 = property class="App"() -> ("App.Kind"=w525:T6)  [unwired: 2 in, 2 out]
        n180 = control-ref of="Current VI Reference"() -> (w519:refnum<vi>)
        n181 = Not(x=w526) -> (.not. x?=w523:bool)
        n182 = Equal?(x=w525, y=T6."Run Time System" ("Application:Kind")) -> (x = y?=w522:bool)
        n183 = Or(x=w523, y=w522) -> (x .or. y?=w520:bool)
        n184 = Bundle By Name(cluster=w521, "Core.Current VI Reference"=w519, "Core.Close Panel on Exit?"=w520) -> (w528:T12)
      }
      frame "Mass Compile Self" {
        w533 = FALSE  # Allow self mass compile
        # "Installed beneath LabVIEW?"
        # "child path?"
        # "Do not delete, rename, or modify this frame.\n(this is used to determine panel behavior on exit)"
        n185 = call <vilib>:"Application Directory.vi"() -> ("Application Directory"=w536:path)
        n186 = call-poly <userlib>:"Build Path__ogtk.vi"("name or relative path"=path[] [path "resource/dialog/QuickDrop/plugins/JKI State Machine Helper__JKI_State_Machine_Helper.vi", path "resource/plugins/PopupMenus/edit time panel and diagram/JKI SM Helper.llb", path "resource/dialog/QuickDrop/plugins/JKI State Machine API", path "resource/dialog/QuickDrop/plugins/_JKI State Machine Helper"], "base path"=w536) -> ("appended path"=w534:path[])
        n187 = call <vilib>:"Application Directory.vi"() -> ("Application Directory"=w531:path)
        n188 = Current VI's Path() -> (path=w530:path)
        n189 = call "Is Child Path -- JKI State Machine Editor.vi"("Path"=w530, "Parent Directory"=w531) -> ("is Child Path?"=w529:bool)
        n190 = Or(x=w533, y=w529) -> (x .or. y?=w532:bool)
        n191 = case shown="True" w532 {
          tunnel: w534 -> [_ w540]
          frame False {
          }
          frame True {
            n192 = call "Mass Compile LabVIEW Tool.vi"("Product Folders"=w540, "Product Name"="JKI State Machine Editor") -> ()  [unwired: 8 in, 2 out]
          }
        }
      }
      frame "Error Handler" {
        w559 = i32[] [1055, 1026]  # Errors signaling shutdown (invalid references, etc.)
        # "Clear Errors"
        # "Clear Errors if Known Error Signaling a Need to Shutdown"
        # "Error Dialog"
        # "Handle any errors here.\nYou can also output any states to clean-up after errors occur"
        n193 = Unbundle By Name(w554) -> ("code"=w556:i32)
        n194 = Search 1D Array(1D array=w559, element=w556) -> (index of element=w558:i32)  [unwired: 1 out]
        n195 = Greater Or Equal To 0?(x=w558) -> (x >= 0?=w555:bool)
        n196 = call <vilib>:"Clear Errors.vi"("error in (no error)"=w554) -> ("error out"=w553:errorcluster)  [unwired: 6 out]
        n197 = Select(t=w553, s=w555, f=w554) -> (s? t:f=w552:errorcluster)
        n198 = Unbundle By Name(w548) -> ("Undo Transaction"=w542:bool)
        n199 = call <vilib>:"Simple Error Handler.vi"("error in (no error)"=w552) -> ("error out"=w551:errorcluster)  [unwired: 4 in, 4 out]
        n200 = Select(t="Macro: Exit", s=w555, f="") -> (s? t:f=w547:string)
        n201 = call <vilib>:"Clear Errors.vi"("error in (no error)"=w551) -> ("error out"=w550:errorcluster)  [unwired: 6 out]
        n202 = Select(t="Script: fail undo", s=w542, f="") -> (s? t:f=w543:string)
        n203 = call <vilib>:"Add State(s) to Queue__jki_lib_state_machine.vi"("State(s) in Front (\"\")"=w547, "State(s) at Back (\"\")"=w543) -> ("States Out"=w546:string)  [unwired: 1 in, 12 out]
      }
      frame "Exit" {
        # "Do not put any code in this frame.\n(No errors that occur here will be handled.)"
      }
      frame "---------- Data ----------" {
        # "Do not put any code in this frame.\n(It is a separator no-op. You can make a copy of this frame to create a new Data frame)"
      }
      frame "Data: Initialize" {
        w567 = -1  # Top Row Index
        w568 = TRUE  # Undo Transaction
        w573 = StructureTypes."CaseStructure"  # Structure Type
        w578 = -1  # NavIndex
        w579 = refnum<vi>[] []  # NavHist
        w583 = ""  # TempString
        w585 = ""  # CaseStrVIName
        w586 = ""  # SectHdr
        w587 = "----------"  # TreeSectHdrs
        w593 = T11 {"Left"=0, "Top"=0, "Right"=0, "Bottom"=0}  # Display:Primary Workspace
        w595 = ""  # Top Row Tag
        w596 = ""  # tag
        w597 = u32 0  # SelectedCase
        w600 = 0  # DisplayedItems
        w601 = string[] []  # FrameNames
        w604 = T13 {"Current VI Reference"=refnum, "Close Panel on Exit?"=FALSE}  # Core
        w582 = FALSE  # Ctrl?
        w584 = FALSE  # Activating
        w594 = refnum<vi> refnum  # CaseStrVI Ref
        w581 = refnum<vi> refnum  # StructRef
        w602 = FALSE  # InBounds
        w603 = FALSE  # Indent?
        # "screen size"
        n204 = control-ref of="This VI"() -> (w569:refnum<vi>)
        n205 = control-ref of="Cases"() -> (w598:refnum<vi>)
        n206 = local read "SelList[]"() -> (w572:refnum<vi>[])
        n207 = Index Array(array=w572) -> (element=w571:refnum<vi>)  [unwired: 1 in]
        n208 = call "Check Is Helper Already Running (Get Queue) -- Wrapper.vi"("Create? (F: Check)"=TRUE, "Helper VI Ref In (if Creating)"=w569, "GObject in"=w571) -> ()  [unwired: 5 in, 4 out]
        n209 = Open Application Reference(8:w589) -> (0:w591:errorcluster, 3:w592:refnum<vi>)  [unwired: 3 in]
        n210 = property class="App"(reference=w592, error in=w591) -> (error out=w590:errorcluster, "Disp.WkSpace"=w588:T11)  [unwired: 1 out]
        n211 = property class="VI"(reference="Active VI Ref") -> ("Name"=w577:string)  [unwired: 1 in, 2 out]
        n212 = Close Reference(reference=w592, error in (no error)=w590) -> (error out=w576:errorcluster)
        n213 = Bundle("Core"=w604, "Indent?"=w603, "InBounds"=w602, "Activating"=w584, "FrameNames"=w601, "tag"=w596, "Top Row Tag"=w595, "TreeSectHdrs"=w587, "SectHdr"=w586, "CaseStrVIName"=w585, "TempString"=w583, "DisplayedItems"=w600, "SelectedCase"=w597, "Display:Primary Workspace"=w593, "Cases"=w598, "StructRef"=w581, "CaseStrVI Ref"=w594, "Ctrl?"=w582, "NavHist"=w579, "NavIndex"=w578, "Structure Type"=w573, "Undo Transaction"=w568, "Top Row Index"=w567) -> (w605:T12)  [unwired: 1 out]
        n214 = Bundle By Name(cluster=w605, "CaseStrVIName"=w577, "CaseStrVI Ref"="Active VI Ref", "Display:Primary Workspace"=w588) -> (w599:T12)
        n215 = property class="VI"(error in=w576, "Front Panel.Title"=w577) -> (error out=w575:errorcluster)  [unwired: 1 in, 1 out]
      }
      frame "Data: get section header" {
        w611 = TRUE ("replace all? (F)")
        n216 = Unbundle By Name(w617) -> ("TreeSectHdrs"=w607:string, "FrameNames"=w606:string[], "tag"=w609:string)
        n217 = while {
          tunnel: w606 -> [w621] mode=indexing
          tunnel: w609 -> [w627]
          tunnel: w607 -> [w624]
          shift-right: [w623] -> w613
          shift-left: "" -> [w622]
          stop <- w620 stop-if-true
          n218 = Equal?(x=w621, y=w627) -> (x = y?=w620:bool)
          n219 = Match Pattern(string=w621, regular expression=w624) -> (offset past match=w626:i32)  [unwired: 4 out]
          n220 = Less Than 0?(x=w626) -> (x < 0?=w625:bool)
          n221 = Select(t=w622, s=w625, f=w621) -> (s? t:f=w623:string)
        }
        n222 = Search and Replace String(replace all?=w611, input string=w613, search string="\"") -> (result string=w612:string)  [unwired: 1 in, 7 out]
        n223 = Search and Replace String(replace all?=w611, input string=w612, search string=w607) -> (result string=w614:string)  [unwired: 1 in, 7 out]
        n224 = call <vilib>:"Trim Whitespace.vi"("string"=w614) -> ("trimmed string"=w608:string)  [unwired: 1 in]
        n225 = Bundle By Name(cluster=w617, "SectHdr"=w608) -> (w616:T12)
      }
      frame "Data: get drop section hdr" {
        # "Get the index of the frame before"
        n226 = Unbundle By Name(w633) -> ("FrameNames"=w631:string[])
        n227 = property on="Cases" class="Tree (strict)"() -> ("All Tags"=w632:string[])  [unwired: 2 in, 2 out]
        n228 = while {
          tunnel: w631 -> [w641]
          tunnel: w632 -> [w640] mode=indexing
          tunnel: [w636] -> w630
          i -> [w637]
          stop <- w638 stop-if-true
          n229 = Search 1D Array(1D array=w641, element=w640) -> (index of element=w639:i32)  [unwired: 1 out]
          n230 = Decrement(x=w637) -> (x-1=w636:i32)
          n231 = Less Than 0?(x=w639) -> (x < 0?=w638:bool)
        }
        n232 = Index Array(array=w631, index=w630) -> (element=w628:string)
        n233 = Bundle By Name(cluster=w633, "tag"=w628) -> (w629:T12)
      }
      frame "Data: Cleanup" {
        # "Cleanup any data and references, here.\n(this is called automatically, by the Macro: Exit)"
        n234 = Unbundle By Name(w645) -> ("Core.Current VI Reference"=w646:refnum<vi>)
        n235 = Close Reference(reference=w646, error in (no error)=w643) -> (error out=w642:errorcluster)
      }
      frame "---------- UI ----------" {
        # "Do not put any code in this frame.\n(It is a separator no-op. You can make a copy of this frame to create a new UI frame)"
      }
      frame "UI: Initialize" {
        w653 = T14."Disabled and Grayed Out" ("Disabled")
        # "Initialize the User Interface, here.\n(this is called automatically, by the Macro: Init)"
        n236 = property on="Back" class="Bool"("DisabledEnum"=w653) -> ()  [unwired: 2 in, 2 out]
        n237 = property on="Forward" class="Bool"("DisabledEnum"=w653) -> ()  [unwired: 2 in, 2 out]
        n238 = property on="Clear History" class="Bool"("DisabledEnum"=w653) -> ()  [unwired: 2 in, 2 out]
        n239 = property on="Search Icon" class="Bool (strict)"("Visible"=TRUE) -> ()  [unwired: 2 in, 2 out]
        n240 = property on="Clear Search" class="Bool (strict)"("Visible"=FALSE) -> ()  [unwired: 2 in, 2 out]
        n241 = local write "Search"("") -> ()
      }
      frame "UI: Update" {
        w663 = T14."Enabled" ("Disabled")
        w664 = T14."Disabled and Grayed Out" ("Disabled")
        # "Initialize the User Interface, here.\n(this is called automatically, by the Macro: Init)"
        n242 = Unbundle By Name(w670) -> ("NavIndex"=w662:i32, "NavHist"=w660:refnum<vi>[])
        n243 = Array Size(array=w660) -> (size(s)=w661:i32)
        n244 = Increment(x=w662) -> (x+1=w659:i32)
        n245 = Equal?(x=0, y=w662) -> (x = y?=w666:bool)
        n246 = Equal?(x=w661, y=w659) -> (x = y?=w658:bool)
        n247 = Empty Array?(array=w660) -> (empty?=w669:bool)
        n248 = Select(t=w664, s=w669, f=w663) -> (s? t:f=w668:T14)
        n249 = Select(t=w664, s=w666, f=w663) -> (s? t:f=w665:T14)
        n250 = Select(t=w664, s=w658, f=w663) -> (s? t:f=w657:T14)
        n251 = property on="Back" class="Bool"("DisabledEnum"=w665) -> ()  [unwired: 2 in, 2 out]
        n252 = property on="Forward" class="Bool"("DisabledEnum"=w657) -> ()  [unwired: 2 in, 2 out]
        n253 = property on="Clear History" class="Bool"("DisabledEnum"=w668) -> ()  [unwired: 2 in, 2 out]
      }
      frame "UI: Front Panel State" {
        # "Set Front Panel Open or Closed\n(Usage: \"UI: Front Panel State >> Open|Close\")"
        n254 = Unbundle By Name(w676) -> ("Core.Current VI Reference"=w675:refnum<vi>)
        n255 = case shown="\"Open\", Default" w673 {
          tunnel: w678 -> [w682 w695]
          tunnel: [w684 w696] -> w677
          tunnel: w675 -> [w683 w693]
          frame "Open", Default {
            n256 = property class="VI"(reference=w683, error in=w682) -> (reference out=w680:refnum<vi>, error out=w681:errorcluster, "Front Panel.Open"=w679:bool)
            n257 = case shown="False" w679 {
              tunnel: [w687 w690] -> w684
              tunnel: w681 -> [w686 w690]
              tunnel: w680 -> [w685 _]
              frame False {
                n258 = invoke class="VI" method="FP.Open"(reference=w685, error in=w686, "Activate"=TRUE, "State"=T5."Standard") -> (error out=w687:errorcluster)  [unwired: 1 in, 4 out]
              }
              frame True {
              }
            }
          }
          frame "Close" {
            n259 = property class="VI"(reference=w693, error in=w695) -> (reference out=w692:refnum<vi>, error out=w694:errorcluster, "Front Panel.Open"=w691:bool)
            n260 = case shown="True" w691 {
              tunnel: [w697 w700] -> w696
              tunnel: w694 -> [w697 w699]
              tunnel: w692 -> [_ w698]
              frame False {
              }
              frame True {
                n261 = invoke class="VI" method="FP.Close"(reference=w698, error in=w699) -> (error out=w700:errorcluster)  [unwired: 1 in, 2 out]
              }
            }
          }
        }
      }
      frame "UI: front panel size" {
        # "FP width"
        # "reposition panel"
        # "top = screen bottom - panel height"
        # "left = screen right - panel width"
        # "panel size"
        n262 = Unbundle By Name(w715) -> ("Display:Primary Workspace.Right"=w705:i16, "Display:Primary Workspace.Bottom"=w704:i16, "Core.Current VI Reference"=w706:refnum<vi>)  [unwired: 2 out]
        n263 = property class="VI"(reference=w706, error in=w714) -> (reference out=w702:refnum<vi>, error out=w703:errorcluster, "Front Panel.WinBounds"=w710:T11)
        n264 = Unbundle By Name(w710) -> ("Right"=w711:i16, "Left"=w712:i16)
        n265 = Subtract(x=w711, y=w712) -> (x-y=w707:i16)
        n266 = Subtract(x=w705, y=w707) -> (x-y=w708:i16)
        n267 = Bundle By Name(cluster=w710, "Right"=w705, "Bottom"=w704, "Left"=w708, "Top"=i16 0 ("x-y")) -> (w709:T11)
        n268 = property class="VI"(reference=w702, error in=w703, "Front Panel.WinBounds"=w709) -> (error out=w713:errorcluster)  [unwired: 1 out]
      }
      frame "UI: defer panel updates" {
        n269 = Unbundle By Name(w731) -> ("Core.Current VI Reference"=w730:refnum<vi>)
        n270 = call <vilib>:"Trim Whitespace.vi"("string"=w729) -> ("trimmed string"=w728:string)  [unwired: 1 in]
        n271 = Equal?(x=w728, y="TRUE") -> (x = y?=w717:bool)
        n272 = property class="VI"(reference=w730, error in=w733) -> (error out=w721:errorcluster, "Panel"=w723:refnum<vi>)  [unwired: 1 out]
        n273 = property class="Pnl"(reference=w723, error in=w721) -> (reference out=w722:refnum<vi>, error out=w720:errorcluster, "DeferPanUpdts"=w719:bool)
        n274 = Not Equal?(x=w717, y=w719) -> (x != y?=w718:bool)
        n275 = case "Requested Value is Different than Current Value? Then: Set Property" shown="True" w718 {
          tunnel: [w734 w739] -> w732
          tunnel: [_ w738] -> w724
          tunnel: w722 -> [_ w737]
          tunnel: w720 -> [w734 w736]
          tunnel: w717 -> [_ w735]
          frame False {
            # "No Op"
          }
          frame True {
            n276 = property class="Pnl"(reference=w737, error in=w736, "DeferPanUpdts"=w735) -> (error out=w739:errorcluster)  [unwired: 1 out]
            n277 = case shown="True" w735 {
              tunnel: [_ "UI: defer panel updates >> FALSE" ("State(s) at Back (\"\")")] -> w738
              frame False {
              }
              frame True {
                # "Un-defer updates *after* all states finish"
              }
            }
          }
        }
        n278 = call <vilib>:"Add State(s) to Queue__jki_lib_state_machine.vi"("State(s) in (\"\")"=w726, "State(s) at Back (\"\")"=w724) -> ("States Out"=w725:string)  [unwired: 1 in, 12 out]
      }
      frame "UI: show/hide scroll bar" {
        n279 = Unbundle By Name(w748) -> ("FrameNames"=w746:string[], "Cases"=w747:refnum<vi>)
        n280 = call "ShowHideScrollBar.vi"("error in"=w750, "reference"=w747) -> ("error out"=w749:errorcluster, "Visible?"=w741:bool)  [unwired: 8 out]
        n281 = case shown="False" w741 {
          tunnel: w748 -> [w756 w757]
          tunnel: w746 -> [w755 _]
          tunnel: [w754 w757] -> w745
          tunnel: ["UI: restore position" _] -> w742
          frame False {
            w751 = 0 ("Top Row Index")
            # "Set the position to the top\nif the scroll bar isn't visible."
            n282 = Index Array(array=w755, index=w751) -> (element=w753:string)
            n283 = Bundle By Name(cluster=w756, "Top Row Tag"=w753, "Top Row Index"=w751) -> (w754:T12)
          }
          frame True {
          }
        }
        n284 = call <vilib>:"Add State(s) to Queue__jki_lib_state_machine.vi"("State(s) in Front (\"\")"=w742, "State(s) in (\"\")"=w744) -> ("States Out"=w743:string)  [unwired: 1 in, 12 out]
      }
      frame "UI: collapse/expand tree" {
        # "found"
        n285 = disable-structure shown="Enabled" {
          disable-tunnel: [w775 w784] -> w764
          disable-tunnel: w763 -> [w774 w784]
          disable-tunnel: w762 -> [w773 _]
          disable-tunnel: w761 -> [w772 _]
          frame Disabled {
            n286 = Unbundle By Name(w773) -> ("FrameNames"=w766:string[], "Cases"=w765:refnum<vi>)
            n287 = Equal?(x=w772, y="Expand All") -> (x = y?=w770:bool)
            n288 = invoke class="Tree (strict)" method="Open/Close.Open/Close All"(reference=w765, error in=w774, "Open"=w770) -> (reference out=w769:refnum<vi>, error out=w768:errorcluster)  [unwired: 1 in, 2 out]
            n289 = Index Array(array=w766) -> (element=w771:string)  [unwired: 1 in]
            n290 = case shown="False" w770 {
              tunnel: w768 -> [w782 w783]
              tunnel: [w781 w783] -> w775
              tunnel: w769 -> [w780 _]
              tunnel: w771 -> [w777 _]
              frame False {
                # "Put the first case at\nthe top of the Tree\nso it doesn't collapse\nand hide the stuff\nat the top of the list."
                n291 = Bundle By Name(cluster=cluster{"Node":string, "Column":i32} {"Node"="", "Column"=0} ("Top Left Visible Cell"), "Node"=w777, "Column"=0) -> (w778:cluster{"Node":string, "Column":i32})
                n292 = property class="Tree (strict)"(reference=w780, error in=w782, "TopLeft"=w778) -> (error out=w781:errorcluster)  [unwired: 1 out]
              }
              frame True {
              }
            }
          }
          frame Enabled {
          }
        }
        n293 = call <vilib>:"Add State(s) to Queue__jki_lib_state_machine.vi"("State(s) in Front (\"\")"="UI: show/hide scroll bar", "State(s) in (\"\")"=w759) -> ("States Out"=w758:string)  [unwired: 1 in, 12 out]
      }
      frame "UI: restore position" {
        n294 = disable-structure shown="Enabled" {
          disable-tunnel: w788 -> [w792 _]
          disable-tunnel: w786 -> [w799 _]
          disable-tunnel: [w798 _] -> w785
          frame Enabled {
            n295 = Unbundle By Name(w799) -> ("Top Row Index"=w794:i32, "Cases"=w789:refnum<vi>)
            n296 = property class="Tree (strict)"(reference=w789, error in=w792) -> (reference out=w790:refnum<vi>, error out=w791:errorcluster, "DispItems"=w795:string[])
            n297 = Index Array(array=w795, index=w794) -> (element=w793:string)
            n298 = Empty String/Path?(string/path=w793) -> (empty?=w797:bool)
            n299 = Not(x=w797) -> (.not. x?=w796:bool)
            n300 = case shown="True" w796 {
              tunnel: w791 -> [w800 w807]
              tunnel: [w800 w806] -> w798
              tunnel: w793 -> [_ w802]
              tunnel: w790 -> [_ w801]
              frame False {
              }
              frame True {
                n301 = Bundle By Name(cluster=cluster{"Node":string, "Column":i32} {"Node"="", "Column"=0} ("Top Left Visible Cell"), "Node"=w802, "Column"=0) -> (w803:cluster{"Node":string, "Column":i32})
                n302 = property class="Tree (strict)"(reference=w801, error in=w807, "TopLeft"=w803) -> (error out=w806:errorcluster)  [unwired: 1 out]
              }
            }
          }
          frame Disabled {
          }
        }
      }
      frame "UI: select message" {
        n303 = One Button Dialog(message="Nothing is selected.") -> ()  [unwired: 2 out]
      }
      frame "---------- Macro ----------" {
        # "Do not put any code in this frame.\n(It is a separator no-op. You can make a copy of this frame to create a new Macro frame)"
      }
      frame "Macro: Initialize" {
        w815 = "Data: Initialize\nInitialize Core Data\nUI: Initialize\n\nScript: get CaseStruct Ref\nMacro: process structure\n\nUI: Update\nUI: show/hide scroll bar\nUI: front panel size\nUI: Front Panel State >> Open"  # Data: Initialize Initialize Core Data UI: Initialize  Script: get CaseStruct Ref Macro: process structure  UI: Update UI: show/hide scroll bar UI: front panel size UI: Front Panel State >> Open
        # "Initialization Macro\n(This is called once, when the VI starts)"
        n304 = call <vilib>:"Add State(s) to Queue__jki_lib_state_machine.vi"("State(s) in Front (\"\")"=w815, "State(s) in (\"\")"=w819) -> ("States Out"=w818:string)  [unwired: 1 in, 12 out]
      }
      frame "Macro: process structure" {
        n305 = call <vilib>:"Add State(s) to Queue__jki_lib_state_machine.vi"("State(s) in Front (\"\")"=w820, "State(s) in (\"\")"=w822) -> ("States Out"=w821:string)  [unwired: 13 in]
      }
      frame "Macro: insert" {
        n306 = Search and Replace String(input string="Data: get section header\nScript: begin undo >> insert\nScript: insert frame >> [FRAME]\nScript: end undo", search string="[FRAME]", replace string=w825) -> (result string=w827:string)  [unwired: 5 in, 3 out]
        n307 = call <vilib>:"Add State(s) to Queue__jki_lib_state_machine.vi"("State(s) in Front (\"\")"=w827, "State(s) in (\"\")"=w830) -> ("States Out"=w829:string)  [unwired: 1 in, 12 out]
      }
      frame "Macro: delete" {
        n308 = Search and Replace String(input string=w833, search string="[FRAME]", replace string=w836, error in=w835) -> (result string=w837:string, error out=w834:errorcluster)  [unwired: 4 in, 2 out]
        n309 = call <vilib>:"Add State(s) to Queue__jki_lib_state_machine.vi"("State(s) in Front (\"\")"=w837, "State(s) in (\"\")"=w840) -> ("States Out"=w839:string)  [unwired: 13 in]
      }
      frame "Macro: Select Case" {
        # "Visible frame not the indext we think it should be?"
        n310 = Unbundle By Name(w853) -> ("tag"=w854:string, "StructRef"=w845:refnum<vi>)
        n311 = call "Script - get FrameNames.vi"("error in"=w844, "StructRef"=w845) -> ("error out"=w843:errorcluster, "Frame Names"=w842:string[])  [unwired: 4 in, 4 out]
        n312 = property class="MFStruct"(reference=w845, error in=w843) -> (error out=w852:errorcluster, "VisFrame"=w851:u32)  [unwired: 1 out]
        n313 = Search 1D Array(1D array=w842, element=w854) -> (index of element=w855:i32)  [unwired: 1 out]
        n314 = To Unsigned Long Integer(number=w855) -> (unsigned 32bit integer=w850:u32)
        n315 = Not Equal?(x=w850, y=w851) -> (x != y?=w849:bool)
        n316 = Search and Replace String(input string="Script: begin undo >> Visible Frame Changed\nScript: select case\nScript: end undo\n//Script: do undo", search string="[FRAME]", replace string=w857, error in=w852) -> (result string=w847:string, error out=w856:errorcluster)  [unwired: 4 in, 2 out]
        n317 = Select(t=w847, s=w849, f="") -> (s? t:f=w846:string)
        n318 = call <vilib>:"Add State(s) to Queue__jki_lib_state_machine.vi"("State(s) in Front (\"\")"=w846, "State(s) in (\"\")"=w861) -> ("States Out"=w860:string)  [unwired: 13 in]
      }
      frame "Macro: update list" {
        n319 = call <vilib>:"Add State(s) to Queue__jki_lib_state_machine.vi"("State(s) in Front (\"\")"=w862, "State(s) in (\"\")"=w864) -> ("States Out"=w863:string)  [unwired: 1 in, 12 out]
      }
      frame "Macro: process drag-copy" {
        n320 = call <vilib>:"Add State(s) to Queue__jki_lib_state_machine.vi"("State(s) in Front (\"\")"="Data: get drop section hdr\nData: get section header\nScript: process drag-copy\nScript: select case" ("message"), "State(s) in (\"\")"=w870) -> ("States Out"=w869:string)  [unwired: 1 in, 12 out]
      }
      frame "Macro: sort list" {
        n321 = call <vilib>:"Add State(s) to Queue__jki_lib_state_machine.vi"("State(s) in Front (\"\")"="Script: begin undo >> sort\nScript: sort list\nScript: end undo\nMacro: update list\nUI: collapse/expand tree >> Expand All", "State(s) in (\"\")"=w874) -> ("States Out"=w873:string)  [unwired: 1 in, 12 out]
      }
      frame "Macro: rename" {
        n322 = Search and Replace String(input string=w877, search string="[FRAME]", replace string=w878, error in=w882) -> (result string=w880:string, error out=w881:errorcluster)  [unwired: 4 in, 2 out]
        n323 = call <vilib>:"Add State(s) to Queue__jki_lib_state_machine.vi"("State(s) in Front (\"\")"=w880, "State(s) in (\"\")"=w885) -> ("States Out"=w884:string)  [unwired: 1 in, 12 out]
      }
      frame "Macro: duplicate" {
        n324 = Search and Replace String(input string="Data: get section header\nScript: begin undo >> rename\nScript: duplicate case >> [FRAME]\nScript: end undo\nMacro: update list", search string="[FRAME]", replace string=w890, error in=w889) -> (result string=w886:string, error out=w888:errorcluster)  [unwired: 4 in, 2 out]
        n325 = call <vilib>:"Add State(s) to Queue__jki_lib_state_machine.vi"("State(s) in Front (\"\")"=w886, "State(s) in (\"\")"=w893) -> ("States Out"=w892:string)  [unwired: 1 in, 12 out]
      }
      frame "Macro: Add Dynamic Events" {
        n326 = call <vilib>:"Add State(s) to Queue__jki_lib_state_machine.vi"("State(s) in Front (\"\")"=w895, "State(s) in (\"\")"=w898) -> ("States Out"=w897:string)  [unwired: 1 in, 12 out]
      }
      frame "Macro: Find Callers" {
        n327 = Search and Replace String(input string="Script: Find Callers >> [FRAME]", search string="[FRAME]", replace string=w904, error in=w903) -> (result string=w900:string, error out=w902:errorcluster)  [unwired: 4 in, 2 out]
        n328 = call <vilib>:"Add State(s) to Queue__jki_lib_state_machine.vi"("State(s) in Front (\"\")"=w900, "State(s) in (\"\")"=w907) -> ("States Out"=w906:string)  [unwired: 1 in, 12 out]
      }
      frame "Macro: drop state name" {
        n329 = call <vilib>:"Add State(s) to Queue__jki_lib_state_machine.vi"("State(s) in Front (\"\")"="Script: begin undo >> drop\nScript: drop state name\nScript: end undo" ("t"), "State(s) in (\"\")"=w911) -> ("States Out"=w910:string)  [unwired: 13 in]
      }
      frame "Macro: append string" {
        n330 = call <vilib>:"Add State(s) to Queue__jki_lib_state_machine.vi"("State(s) in Front (\"\")"="Script: begin undo >> append\nScript: append string\nScript: end undo" ("t"), "State(s) in (\"\")"=w916) -> ("States Out"=w915:string)  [unwired: 13 in]
      }
      frame "Macro: copy frame" {
        n331 = Match Pattern(string=w923, regular expression=",") -> (before substring=w921:string, after substring=w920:string)  [unwired: 1 in, 2 out]
        n332 = Format Into String(format string="Script: begin undo >> copy\nScript: copy frame >> %s,%s\nScript: end undo", w921, w920) -> (resulting string=w919:string)  [unwired: 2 in, 1 out]
        n333 = call <vilib>:"Add State(s) to Queue__jki_lib_state_machine.vi"("State(s) in Front (\"\")"=w919, "State(s) in (\"\")"=w926) -> ("States Out"=w925:string)  [unwired: 13 in]
      }
      frame "Macro: Exit" {
        # "Exit Macro\n(This is called once, when the VI exits)"
        n334 = call <vilib>:"Add State(s) to Queue__jki_lib_state_machine.vi"("State(s) in Front (\"\")"="UI: Front Panel State >> Close\nData: Cleanup\nExit", "State(s) in (\"\")"=w933) -> ("States Out"=w932:string)  [unwired: 1 in, 12 out]
      }
      frame "---------- Navigate ----------" {
      }
      frame "Navigate: Add" {
        n335 = Unbundle By Name(w945) -> ("StructRef"=w944:refnum<vi>)
        n336 = call "Script - get FrameNames.vi"("error in"=w943, "StructRef"=w944) -> ("error out"=w942:errorcluster, "Frame Names"=w941:string[], "Frames[]"=w939:refnum<vi>[])  [unwired: 4 in, 3 out]
        n337 = Search 1D Array(1D array=w941, element=w937) -> (index of element=w940:i32)  [unwired: 1 in]
        n338 = Index Array(array=w939, index=w940) -> (element=w938:refnum<vi>)
        n339 = in-place {
          in-place-border: w938 -> [w953]
          in-place-border: w937 -> [w948]
          n340 = in-place-cluster #1(w945) -> ("NavHist"=w951:refnum<vi>[], "NavIndex"=w952:i32)  [unwired: 1 out]
          n341 = Increment(x=w952) -> (x+1=w950:i32)
          n342 = Reshape Array(w951, w950) -> (w949:refnum<vi>[])
          n343 = Increment(x=w952) -> (x+1=w955:i32)
          n344 = Build Array (concatenate)(w949, w953) -> (w954:refnum<vi>[])
          n345 = in-place-cluster #1("NavHist"=w954, "NavIndex"=w955, "tag"=w948) -> (w946:T12)
        }
      }
      frame "Navigation: Clear History" {
        n346 = Unbundle By Name(w961) -> ("StructRef"=w959:refnum<vi>)
        n347 = call "Script - get FrameNames.vi"("error in"=w958, "StructRef"=w959) -> ("error out"=w957:errorcluster, "Visible Frame"=w956:refnum<vi>)  [unwired: 4 in, 4 out]
        n348 = Build Array(w956) -> (w962:refnum<vi>[])
        n349 = Bundle By Name(cluster=w961, "NavHist"=w962, "NavIndex"=0) -> (w960:T12)
      }
      frame "---------- Scripting ----------" {
      }
      frame "Script: begin undo" {
        n350 = Unbundle By Name(w973) -> ("CaseStrVI Ref"=w970:refnum<vi>)
        n351 = Bundle By Name(cluster=w973, "Undo Transaction"=TRUE) -> (w969:T12)
        n352 = invoke class="VI" method="Transaction.Begin Undo"(reference=w970, error in=w971, "Name"=w972) -> (error out=w974:errorcluster)  [unwired: 1 in, 3 out]
      }
      frame "Script: get CaseStruct ref" {
        w985 = refnum<vi> refnum  # MultiFrameStructure
        w989 = refnum<vi> refnum  # CaseStructure
        w990 = refnum<vi> refnum  # EventStructure
        # "I get the Active VI Ref from the RCF because I\nwant to implement Undo and I think I need that.\n\nGet the reference to the Case Structure here."
        n353 = Unbundle By Name(w997) -> ("CaseStrVI Ref"=w992:refnum<vi>)
        n354 = property class="VI"(reference=w992, error in=w993) -> (error out=w977:errorcluster, "Diagram"=w996:refnum<vi>)  [unwired: 1 out]
        n355 = property class="TopLvlDiag" props=["SelList[]"](reference=w996, error in=w977) -> (error out=w984:errorcluster)  [unwired: 2 out]
        n356 = Index Array(array="SelList[]") -> (element=w982:refnum<vi>)  [unwired: 1 in]
        n357 = To More Specific Class(target class=w990, reference=w982, error in=w984) -> (error out=w988:errorcluster)  [unwired: 1 out]
        n358 = To More Specific Class(target class=w989, reference=w982, error in=w984) -> (error out=w978:errorcluster)  [unwired: 1 out]
        n359 = To More Specific Class(target class=w985, reference=w982, error in=w984) -> (specific class reference=w981:refnum<vi>, error out=w983:errorcluster)
        n360 = property class="MFStruct"(reference=w981, error in=w983) -> (reference out=w980:refnum<vi>, error out=w991:errorcluster, "OwningVI"=w994:refnum<vi>)
        n361 = call <vilib>:"Clear Errors.vi"("error in (no error)"=w978) -> ()  [unwired: 6 in, 1 out]
        n362 = Select(t=StructureTypes."CaseStructure" ("Structure Type"), s=w988, f=StructureTypes."EventStructure" ("Structure Type")) -> (s? t:f=w979:T7)
        n363 = Bundle By Name(cluster=w997, "Structure Type"=w979, "StructRef"=w980, "CaseStrVI Ref"=w994) -> (w995:T12)
      }
      frame "Script: get FrameNames" {
        w1007 = 1 items=["no exception", "cancel error on match", "set error on match"] ("[exception action] (none:0)")
        # "Why, oh why, did I put this here?\nI wish I commented it back then..."
        n364 = Unbundle By Name(w1013) -> ("Cases"=w1002:refnum<vi>, "StructRef"=w1005:refnum<vi>)
        n365 = call "Script - get FrameNames.vi"("error in"=w1016, "StructRef"=w1005) -> ("error out"=w1012:errorcluster, "Visible Frame Index"=w1003:u32, "Frame Names"=w1004:string[])  [unwired: 4 in, 3 out]
        n366 = property class="Tree (strict)"(reference=w1002, error in=w1012) -> (error out=w1010:errorcluster, "DispItems"=w1001:string[], "TopLeft"=w1009:T10)  [unwired: 1 out]
        n367 = Unbundle By Name(w1009) -> ("Node"=w1000:string)
        n368 = call <vilib>:"General Error Handler.vi"("error in (no error)"=w1010, "[exception action] (none:0)"=w1007, "[exception code]"=1136) -> ("error out"=w1008:errorcluster)  [unwired: 1 in, 11 out]
        n369 = Search 1D Array(1D array=w1001, element=w1000) -> (index of element=w999:i32)  [unwired: 1 in]
        n370 = Bundle By Name(cluster=w1013, "FrameNames"=w1004, "SelectedCase"=w1003, "Top Row Tag"=w1000, "Top Row Index"=w999) -> (w1011:T12)
        n371 = call <vilib>:"Add State(s) to Queue__jki_lib_state_machine.vi"("State(s) in (\"\")"=w1015) -> ("States Out"=w1014:string)  [unwired: 2 in, 12 out]
      }
      frame "Script: check indent" {
        # "I only want to indent if the states\nin this Case Structure have section\nseparators (like the JKI SM).  Otherwise\nI'll put all items in the first col of the Tree."
        n372 = Unbundle By Name(w1025) -> ("FrameNames"=w1023:string[], "Core.Current VI Reference"=w1022:refnum<vi>)
        n373 = for {
          tunnel: w1023 -> [w1033] mode=indexing
          shift-right: [w1029] -> w1028
          shift-left: FALSE -> [w1030]
          n374 = Match Pattern(string=w1033, regular expression="-------") -> (offset past match=w1032:i32)  [unwired: 4 out]
          n375 = Greater Or Equal To 0?(x=w1032) -> (x >= 0?=w1031:bool)
          n376 = Or(x=w1031, y=w1030) -> (x .or. y?=w1029:bool)
        }
        n377 = property class="VI"(reference=w1022, error in=w1019) -> (error out=w1020:errorcluster, "Panel"=w1021:refnum<vi>)  [unwired: 1 out]
        n378 = property class="Pnl"(reference=w1021, error in=w1020, "DeferPanUpdts"=TRUE ("Defer Panel Updates")) -> (error out=w1018:errorcluster)  [unwired: 1 out]
        n379 = Bundle By Name(cluster=w1025, "Indent?"=w1028) -> (w1024:T12)
      }
      frame "Script: populate tree" {
        # "DO NOT CALL THIS FRAME DIRECTLY\nCALL \"Macro: update list\" instead, which will defer panel updates and other things"
        n380 = Unbundle By Name(w1040) -> ("Indent?"=w1045:bool, "FrameNames"=w1036:string[], "TreeSectHdrs"=w1038:string, "Cases"=w1044:refnum<vi>)
        n381 = invoke class="Tree (strict)" method="Edit Tree Items.Delete"(reference=w1044, error in=w1043, "Delete Children"=TRUE ("Delete Children?")) -> (reference out=w1047:refnum<vi>, error out=w1048:errorcluster)  [unwired: 2 in, 3 out]
        n382 = call "JKI SM EDITOR - quick filter list.vi"("quick filter text"="Search", "States"=w1036) -> ("States quick-filtered"=w1035:string[])  [unwired: 11 in, 2 out]
        n383 = for {
          tunnel: w1038 -> [w1055]
          tunnel: w1045 -> [w1054]
          tunnel: w1035 -> [w1053] mode=indexing
          shift-right: [w1057] -> w1050
          shift-left: w1047 -> [w1067]
          shift-right: [w1056] -> w1051
          shift-left: w1048 -> [w1066]
          i -> [w1060]
          # "Don't indent the first case."
          # "Fill the Tree"
          n384 = Match Pattern(string=w1053, regular expression=w1055) -> (offset past match=w1065:i32)  [unwired: 4 out]
          n385 = Less Than 0?(x=w1065) -> (x < 0?=w1064:bool)
          n386 = Not Equal To 0?(x=w1060) -> (x != 0?=w1058:bool)
          n387 = Compound Arithmetic op=AND(w1054, w1064, w1058) -> (w1059:bool)
          n388 = Select(t=1 ("New Item Indentation"), s=w1059, f=0 ("New Item Indentation")) -> (s? t:f=w1061:i32)
          n389 = invoke class="Tree (strict)" method="Edit Tree Items.Add Item to End"(reference=w1067, error in=w1066, "Left Cell"=w1053, "Child Tag"=w1053, "Item Indent"=w1061) -> (reference out=w1057:refnum<vi>, error out=w1056:errorcluster)  [unwired: 3 in, 6 out]
        }
        n390 = property class="Tree (strict)"(reference=w1050, error in=w1051) -> (error out=w1042:errorcluster, "DispItems"=w1049:string[])  [unwired: 1 out]
        n391 = Array Size(array=w1049) -> (size(s)=w1052:i32)
        n392 = Bundle By Name(cluster=w1040, "DisplayedItems"=w1052) -> (w1039:T12)
      }
      frame "Script: select case" {
        n393 = Unbundle By Name(w1080) -> ("tag"=w1070:string, "StructRef"=w1075:refnum<vi>)
        n394 = call "Script - get FrameNames.vi"("error in"=w1073, "StructRef"=w1075) -> ("error out"=w1072:errorcluster, "Visible Frame Name"=w1074:string, "Frame Names"=w1071:string[])  [unwired: 4 in, 3 out]
        n395 = Not Equal?(x=w1070, y=w1074) -> (x != y?=w1069:bool)
        n396 = Search 1D Array(1D array=w1071, element=w1070) -> (index of element=w1068:i32)  [unwired: 1 out]
        n397 = Bundle By Name(cluster=w1080, "SelectedCase"=w1068) -> (w1076:T12)
        n398 = case shown="True" w1069 {
          tunnel: [w1082 w1086] -> w1078
          tunnel: w1075 -> [_ w1085]
          tunnel: w1072 -> [w1082 w1084]
          tunnel: w1068 -> [_ w1083]
          frame False {
          }
          frame True {
            n399 = property class="MFStruct"(reference=w1085, error in=w1084, "VisFrame"=w1083) -> (error out=w1086:errorcluster)  [unwired: 1 out]
          }
        }
        n400 = Unbundle By Name(w1078) -> ("code"=w1077:i32)
        n401 = case shown="1" w1077 {
          tunnel: [w1087 w1089 w1090] -> w1079
          tunnel: w1078 -> [w1087 w1088 w1090]
          frame 0, Default {
          }
          frame 1 {
            # "Ignore error after drag/copy operation."
            n402 = call <vilib>:"Clear Errors.vi"("error in (no error)"=w1088) -> ("error out"=w1089:errorcluster)  [unwired: 6 out]
          }
          frame 1055 {
            # "Invalid reference"
          }
        }
      }
      frame "Script: sort list" {
        n403 = Unbundle By Name(w1098) -> ("StructRef"=w1091:refnum<vi>, "FrameNames"=w1093:string[], "TreeSectHdrs"=w1092:string)
        n404 = call "SortAlphabetically.vi"("error in"=w1096, "TreeSectHdrs"=w1092, "FrameNames"=w1093) -> ("error out"=w1095:errorcluster, "Sorted"=w1094:i32[])  [unwired: 7 out]
        n405 = invoke class="MFStruct" method="RearrangeFramesByIdx"(reference=w1091, error in=w1095, "Index Array"=w1094) -> (error out=w1097:errorcluster)  [unwired: 1 in, 3 out]
      }
      frame "Script: Add Dynamic Events" {
        n406 = Unbundle By Name(w1107) -> ("StructRef"=w1102:refnum<vi>)
        n407 = call "Create (From Structure).vi"("error in (no error)"=w1101, "Structure"=w1102) -> ("error out"=w1104:errorcluster, "JKI SM out"=w1106:refnum<class "JKI SM.lvclass">)  [unwired: 8 in]
        n408 = call-dynamic "Add Event Registration Category.vi"("error in (no error)"=w1104, "JKI SM in"=w1106) -> ("error out"=w1103:errorcluster, "JKI SM out"=w1105:refnum<class "JKI SM.lvclass">)  [unwired: 8 in]
        n409 = call "Destroy.vi"("error in (no error)"=w1103, "JKI SM in"=w1105) -> ("error out"=w1100:errorcluster)  [unwired: 9 in]
      }
      frame "Script: delete frame" {
        # "commented this out"
        # "Don't need to do full tree refresh if we delete single item in tree here."
        n410 = Unbundle By Name(w1119) -> ("FrameNames"=w1114:string[], "StructRef"=w1118:refnum<vi>, "Structure Type"=w1111:T7, "Cases"=w1109:refnum<vi>)
        n411 = Empty String/Path?(string/path=w1110) -> (empty?=w1112:bool)
        n412 = case shown="False" w1112 {
          tunnel: w1120 -> [w1142 w1175]
          tunnel: w1118 -> [w1140 _]
          tunnel: w1114 -> [w1138 _]
          tunnel: [w1132 w1175] -> w1113
          tunnel: w1110 -> [w1121 _]
          tunnel: w1111 -> [w1131 _]
          tunnel: w1109 -> [w1122 _]
          frame False {
            # "An unnamed case seems to have the tag \"_1\"; go figure.\nI'll work on this later...  For now, I'll search for an empty\nstring and delete that one (it'll always be the first one."
            # "Find 1st case\nw/o a name"
            n413 = call "Parse State from Frame Name.vi"("Frame or State Name"=w1121) -> ("is a Category Frame?"=w1123:bool, "Category Name"=w1125:string)  [unwired: 6 in, 3 out]
            n414 = Select(t=w1125, s=w1123, f=w1121) -> (s? t:f=w1124:string)
            n415 = Search 1D Array(1D array=w1138, element="") -> (index of element=w1135:i32)  [unwired: 1 out]
            n416 = Search 1D Array(1D array=w1138, element=w1121) -> (index of element=w1133:i32)  [unwired: 1 out]
            n417 = Less Than 0?(x=w1133) -> (x < 0?=w1136:bool)
            n418 = Select(t="", s=w1136, f=w1124) -> (s? t:f=w1129:string)
            n419 = Select(t=w1135, s=w1136, f=w1133) -> (s? t:f=w1134:i32)
            n420 = Select(t="Delete \"%s\" category?" ("format string"), s=w1123, f="Delete %s frame and all callers?\n(use Find Callers if unsure)" ("format string")) -> (s? t:f=w1126:string)
            n421 = Format Into String(format string=w1126, w1129) -> (resulting string=w1141:string)  [unwired: 2 in, 1 out]
            n422 = Two Button Dialog(message=w1141) -> (T button?=w1130:bool)  [unwired: 2 out]
            n423 = case shown="True" w1130 {
              tunnel: w1142 -> [w1143 w1155]
              tunnel: [w1143 w1144] -> w1132
              tunnel: w1140 -> [_ w1154]
              tunnel: w1134 -> [_ w1153]
              tunnel: w1131 -> [_ w1151]
              tunnel: w1129 -> [_ w1150]
              tunnel: w1123 -> [_ w1149]
              tunnel: w1122 -> [_ w1146]
              tunnel: w1121 -> [_ w1147]
              frame False {
              }
              frame True {
                w1148 = FALSE  # Delete Children?
                # "Delete Item"
                n424 = To Unsigned Long Integer(number=w1153) -> (unsigned 32bit integer=w1152:u32)
                n425 = case shown="\"CaseStructure\"" w1151 {
                  tunnel: w1155 -> [w1167 w1173]
                  tunnel: [w1156 w1172] -> w1145
                  tunnel: w1154 -> [w1168 w1171]
                  tunnel: w1152 -> [_ w1170]
                  tunnel: w1151 -> [_ w1169]
                  tunnel: w1150 -> [w1160 _]
                  tunnel: w1149 -> [w1161 _]
                  tunnel: w1147 -> [_ _]
                  frame "CaseStructure" {
                    n426 = Swap Values(12:"", 13:w1161, 14:w1160) -> (1:w1157:string, 3:w1159:string)
                    n427 = call "Create (From Structure).vi"("error in (no error)"=w1167, "Structure"=w1168) -> ("error out"=w1166:errorcluster, "JKI SM out"=w1165:refnum<class "JKI SM.lvclass">)  [unwired: 8 in]
                    n428 = call "Delete State.vi"("Delete Callers? (F: Only Delete Case Structure Frame)"=TRUE, "error in (no error)"=w1166, "State Name"=w1159, "Category (Optional)"=w1157, "JKI SM in"=w1165) -> ("error out"=w1164:errorcluster, "JKI SM out"=w1163:refnum<class "JKI SM.lvclass">)  [unwired: 5 in]
                    n429 = call "Destroy.vi"("error in (no error)"=w1164, "JKI SM in"=w1163) -> ("error out"=w1156:errorcluster)  [unwired: 9 in]
                  }
                  frame "EventStructure" {
                    n430 = call "Script - delete frame.vi"("errorin"=w1173, "Structure Type"=w1169, "Frame Index"=w1170, "StructRef"=w1171) -> ("error out"=w1172:errorcluster)  [unwired: 7 in]
                  }
                }
                n431 = invoke on="Tree: Delete Item" class="Tree (strict)" method="Edit Tree Items.Delete"(reference=w1146, error in=w1145, "tag"=w1147, "Delete Children"=w1148) -> (error out=w1144:errorcluster)  [unwired: 1 in, 4 out]
              }
            }
          }
          frame True {
            n432 = One Button Dialog(message="You need to select a case first.") -> ()  [unwired: 2 out]
          }
        }
        n433 = call <vilib>:"Add State(s) to Queue__jki_lib_state_machine.vi"("State(s) in Front (\"\")"="// Macro: update list" ("State(s) in Front (\"\")"), "State(s) in (\"\")"=w1117) -> ("States Out"=w1116:string)  [unwired: 1 in, 12 out]
      }
      frame "Script: insert frame" {
        n434 = Unbundle By Name(w1188) -> ("Structure Type"=w1178:T7, "FrameNames"=w1181:string[], "StructRef"=w1186:refnum<vi>)
        n435 = call "Parse State from Frame Name.vi"("Frame or State Name"=w1176) -> ("Category Name"=w1177:string)  [unwired: 6 in, 4 out]
        n436 = call "PromptUserWithDefault.vi"("Structure Type"=w1178, "Section"=w1177) -> ("OK"=w1179:bool, "NewTag 2"=w1180:string)  [unwired: 2 in, 6 out]
        n437 = Search 1D Array(1D array=w1181, element=w1176) -> (index of element=w1185:i32)  [unwired: 1 out]
        n438 = case shown="True" w1179 {
          tunnel: w1189 -> [w1190 w1202]
          tunnel: [w1190 w1200] -> w1187
          tunnel: w1186 -> [_ w1201]
          tunnel: w1185 -> [_ w1197]
          tunnel: w1180 -> [_ w1193]
          tunnel: w1181 -> [_ w1195]
          tunnel: w1178 -> [_ w1194]
          tunnel: w1176 -> [_ w1191]
          frame False {
            # "User cancelled the operation."
          }
          frame True {
            n439 = Array Size(array=w1195) -> (size(s)=w1196:i32)
            n440 = Less Than 0?(x=w1197) -> (x < 0?=w1198:bool)
            n441 = Select(t=w1196, s=w1198, f=w1197) -> (s? t:f=w1192:i32)
            n442 = Insert Into Array(array=w1195, index=w1192, new element=w1193) -> (w1199:string[])
            n443 = case shown="\"CaseStructure\"" w1194 {
              tunnel: w1202 -> [w1214 w1224]
              tunnel: w1201 -> [w1211 w1223]
              tunnel: [w1209 w1220] -> w1200
              tunnel: w1199 -> [_ w1219]
              tunnel: w1197 -> [w1210 w1218]
              tunnel: w1194 -> [_ w1215]
              tunnel: w1193 -> [w1203 _]
              tunnel: w1192 -> [_ _]
              tunnel: w1192 -> [_ _]
              tunnel: w1191 -> [w1208 _]
              frame "CaseStructure" {
                n444 = Increment(x=w1210) -> ()  [unwired: 1 out]
                n445 = call "Create (From Structure).vi"("error in (no error)"=w1214, "Structure"=w1211) -> ("error out"=w1213:errorcluster, "JKI SM out"=w1212:refnum<class "JKI SM.lvclass">)  [unwired: 8 in]
                n446 = call "Add New State.vi"("After State (Optional)"=w1208, "error in (no error)"=w1213, "State Name"=w1203, "JKI SM in"=w1212) -> ("error out"=w1205:errorcluster, "JKI SM out"=w1207:refnum<class "JKI SM.lvclass">)  [unwired: 5 in, 1 out]
                n447 = call "Set Visible State.vi"("error in (no error)"=w1205, "State Name"=w1203, "JKI SM in"=w1207) -> ("error out"=w1204:errorcluster, "JKI SM out"=w1206:refnum<class "JKI SM.lvclass">)  [unwired: 7 in]
                n448 = call "Destroy.vi"("error in (no error)"=w1204, "JKI SM in"=w1206) -> ("error out"=w1209:errorcluster)  [unwired: 9 in]
              }
              frame "EventStructure" {
                n449 = To Unsigned Long Integer(number=w1218) -> (unsigned 32bit integer=w1222:u32)
                n450 = invoke class="MFStruct" method="Add Frame"(reference=w1223, error in=w1224, "Reference Frame Index"=w1222, "After? (T)"=FALSE) -> (reference out=w1216:refnum<vi>, error out=w1217:errorcluster)  [unwired: 1 in, 3 out]
                n451 = case shown="\"CaseStructure\"" w1215 {
                  tunnel: [w1225 w1232] -> w1220
                  tunnel: w1219 -> [_ w1231]
                  tunnel: w1217 -> [w1225 w1229]
                  tunnel: w1216 -> [_ w1228]
                  frame "EventStructure" {
                  }
                  frame "CaseStructure" {
                    w1230 = refnum<vi> refnum  # CaseStructure
                    n452 = To More Specific Class(target class=w1230, reference=w1228, error in=w1229) -> (specific class reference=w1227:refnum<vi>, error out=w1226:errorcluster)
                    n453 = property class="CaseSel"(reference=w1227, error in=w1226, "FrameNames"=w1231) -> (error out=w1232:errorcluster)  [unwired: 1 out]
                  }
                }
              }
            }
          }
        }
        n454 = call <vilib>:"Add State(s) to Queue__jki_lib_state_machine.vi"("State(s) in Front (\"\")"="Macro: update list" ("State(s) in Front (\"\")"), "State(s) in (\"\")"=w1184) -> ("States Out"=w1183:string)  [unwired: 1 in, 12 out]
      }
      frame "Script: rename case" {
        n455 = Unbundle By Name(w1236) -> ("Cases"=w1233:refnum<vi>, "Structure Type"=w1241:T7, "StructRef"=w1243:refnum<vi>)
        n456 = call "Parse State from Frame Name.vi"("Frame or State Name"=w1234) -> ("is a Category Frame?"=w1240:bool, "State Name"=w1238:string, "Category Name"=w1239:string, "\"Category: State\" String"=w1237:string)  [unwired: 6 in, 1 out]
        n457 = case shown="\"CaseStructure\", Default" w1241 {
          tunnel: [w1263 w1306] -> w1245
          tunnel: w1239 -> [w1262 _]
          tunnel: w1234 -> [w1261 _]
          tunnel: w1243 -> [w1259 _]
          tunnel: w1242 -> [w1257 w1306]
          tunnel: w1238 -> [w1255 _]
          tunnel: w1240 -> [w1254 _]
          tunnel: w1239 -> [w1252 _]
          tunnel: w1238 -> [w1251 _]
          tunnel: w1237 -> [w1250 _]
          tunnel: w1236 -> [w1249 w1305]
          tunnel: [w1248 w1305] -> w1235
          tunnel: w1234 -> [w1247 _]
          tunnel: w1233 -> [w1246 _]
          frame "CaseStructure", Default {
            w1260 = refnum<vi> refnum  # CaseStructure
            n458 = To More Specific Class(target class=w1260, reference=w1259, error in=w1257) -> (specific class reference=w1258:refnum<vi>, error out=w1256:errorcluster)
            n459 = call "PromptUserWithDefault.vi"("is Category?"=w1254, "Recommended Name (\"\": None)"=w1255, "Section"=w1262) -> ("OK"=w1253:bool, "NewTag 2"=w1264:string)  [unwired: 1 in, 6 out]
            n460 = case shown="True" w1253 {
              tunnel: w1264 -> [_ w1273]
              tunnel: [w1266 w1269] -> w1263
              tunnel: w1261 -> [_ _]
              tunnel: w1258 -> [_ w1285]
              tunnel: w1256 -> [w1266 w1286]
              tunnel: w1252 -> [_ w1284]
              tunnel: w1251 -> [_ w1283]
              tunnel: w1250 -> [_ _]
              tunnel: w1249 -> [w1265 w1274]
              tunnel: [w1265 w1274] -> w1248
              tunnel: w1247 -> [_ _]
              tunnel: w1246 -> [_ w1271]
              frame False {
              }
              frame True {
                # "Throws errors\nJust do a \nMacro: update list"
                n461 = call "Create (From Structure).vi"("error in (no error)"=w1286, "Structure"=w1285) -> ("error out"=w1276:errorcluster, "JKI SM out"=w1278:refnum<class "JKI SM.lvclass">)  [unwired: 8 in]
                n462 = call "Parse State from Frame Name.vi"("Wrap in Quotes? (FALSE)"=TRUE, "Frame or State Name"=w1273) -> ("State Name"=w1281:string, "Category Name"=w1282:string)  [unwired: 5 in, 3 out]
                n463 = call "Get VI Reference.vi"("error in (no error)"=w1276, "JKI SM in"=w1278) -> ("error out"=w1275:errorcluster, "JKI SM out"=w1277:refnum<class "JKI SM.lvclass">)  [unwired: 7 in, 1 out]
                n464 = call-dynamic "Rename State.vi"("Category"=w1284, "State"=w1283, "error in (no error)"=w1275, "New State"=w1281, "New Category (\"\": Use Existing)"=w1282, "JKI SM in"=w1277) -> ("error out"=w1280:errorcluster, "New Frame Names"=w1267:string[], "Old Frame Names"=w1268:string[], "JKI SM out"=w1279:refnum<class "JKI SM.lvclass">)  [unwired: 2 in]
                n465 = call "Destroy.vi"("error in (no error)"=w1280, "JKI SM in"=w1279) -> ("error out"=w1272:errorcluster)  [unwired: 9 in]
                n466 = disable-structure shown="Disabled" {
                  disable-tunnel: w1272 -> [w1293 w1304]
                  disable-tunnel: w1271 -> [w1292 _]
                  disable-tunnel: [w1291 w1304] -> w1269
                  disable-tunnel: w1268 -> [w1290 _]
                  disable-tunnel: w1267 -> [w1289 _]
                  frame Disabled {
                    # "Don't need to do full tree refresh if we rename single item in tree here."
                    n467 = call-poly <userlib>:"Trim Whitespace__ogtk.vi"("String in"=w1290) -> ("String out"=w1288:string[])  [unwired: 6 in]
                    n468 = call-poly <userlib>:"Trim Whitespace__ogtk.vi"("String in"=w1289) -> ("String out"=w1287:string[])  [unwired: 6 in]
                    n469 = for "Update Tree with Renames" {
                      shift-right: [w1298] -> w1291
                      shift-left: w1293 -> [w1303]
                      shift-right: [w1296] -> _
                      shift-left: w1292 -> [w1300]
                      tunnel: w1288 -> [w1295] mode=indexing
                      tunnel: w1287 -> [w1294] mode=indexing
                      w1302 = 0  # Left Text
                      # "Rename tags"
                      # "Rename Item Displayed Text"
                      n470 = invoke on="Tree Rename Item Tag" class="Tree (strict)" method="Edit Tree Items.Set Tag"(reference=w1300, error in=w1303, "tag"=w1295, "new tag"=w1294) -> (reference out=w1297:refnum<vi>, error out=w1299:errorcluster, "Edit Tree Items:Set Tag"=w1301:string)  [unwired: 1 in, 2 out]
                      n471 = property class="Tree (strict)"(reference=w1297, error in=w1299, "Active Item Tag"=w1301, "ActiveColNum"=w1302, "Cell String"=w1301) -> (reference out=w1296:refnum<vi>, error out=w1298:errorcluster)
                    }
                  }
                  frame Enabled {
                  }
                }
              }
            }
          }
          frame "EventStructure" {
            # "renaming cases doesn't apply to Event Structures"
          }
        }
      }
      frame "Script: duplicate case" {
        n472 = Unbundle By Name(w1319) -> ("Structure Type"=w1311:T7, "FrameNames"=w1318:string[], "StructRef"=w1313:refnum<vi>)
        n473 = call "Parse State from Frame Name.vi"("Frame or State Name"=w1307) -> ("is a Category Frame?"=w1308:bool, "State Name"=w1309:string, "Category Name"=w1310:string)  [unwired: 6 in, 2 out]
        n474 = case shown="\"CaseStructure\", Default" w1311 {
          tunnel: w1318 -> [w1340 w1383]
          tunnel: [w1336 w1371] -> w1317
          tunnel: w1310 -> [w1325 _]
          tunnel: [w1335 ""] -> w1314
          tunnel: w1307 -> [w1334 w1381]
          tunnel: w1313 -> [w1332 w1379]
          tunnel: w1312 -> [w1330 w1377]
          tunnel: w1309 -> [w1328 _]
          tunnel: w1308 -> [w1320 _]
          frame "CaseStructure", Default {
            w1333 = refnum<vi> refnum  # CaseStructure
            n475 = Swap Values(12:"", 13:w1320, 14:" (copy)" ("string")) -> (1:w1321:string, 3:w1322:string)
            n476 = To More Specific Class(target class=w1333, reference=w1332, error in=w1330) -> (specific class reference=w1331:refnum<vi>, error out=w1329:errorcluster)
            n477 = Concatenate Strings(w1328, w1322) -> (w1327:string)
            n478 = Concatenate Strings(w1325, w1321) -> (w1326:string)
            n479 = Search 1D Array(1D array=w1340, element=w1334) -> (index of element=w1339:i32)  [unwired: 1 out]
            n480 = call "PromptUserWithDefault.vi"("is Category?"=w1320, "Recommended Name (\"\": None)"=w1327, "Section"=w1326) -> ("OK"=w1337:bool, "NewTag 2"=w1338:string)  [unwired: 1 in, 6 out]
            n481 = case shown="True" w1337 {
              tunnel: w1340 -> [_ w1346]
              tunnel: w1339 -> [_ w1344]
              tunnel: w1338 -> [_ w1345]
              tunnel: w1329 -> [w1341 w1349]
              tunnel: [w1341 w1343] -> w1336
              tunnel: w1331 -> [_ w1348]
              tunnel: [_ ""] -> w1335
              tunnel: w1334 -> [_ w1342]
              frame False {
              }
              frame True {
                n482 = disable-structure shown="Enabled" {
                  disable-tunnel: w1349 -> [w1359 w1368]
                  disable-tunnel: w1348 -> [w1358 w1369]
                  disable-tunnel: w1346 -> [w1357 _]
                  disable-tunnel: w1345 -> [w1356 w1360]
                  disable-tunnel: w1344 -> [w1355 _]
                  disable-tunnel: [w1351 w1362] -> w1343
                  disable-tunnel: w1342 -> [_ w1370]
                  frame Disabled {
                    n483 = Increment(x=w1355) -> (x+1=w1350:i32)
                    n484 = invoke class="CaseSel" method="Duplicate Frame"(reference=w1358, error in=w1359, "Frame Index"=w1355) -> (reference out=w1354:refnum<vi>, error out=w1352:errorcluster)  [unwired: 1 in, 2 out]
                    n485 = Insert Into Array(array=w1357, index=w1350, new element=w1356) -> (w1353:string[])
                    n486 = property class="CaseSel"(reference=w1354, error in=w1352, "FrameNames"=w1353) -> (error out=w1351:errorcluster)  [unwired: 1 out]
                  }
                  frame Enabled {
                    n487 = call "Create (From Structure).vi"("error in (no error)"=w1368, "Structure"=w1369) -> ("error out"=w1367:errorcluster, "JKI SM out"=w1366:refnum<class "JKI SM.lvclass">)  [unwired: 8 in]
                    n488 = call-dynamic "Duplicate State.vi"("State to Duplicate"=w1370, "error in (no error)"=w1367, "New State"=w1360, "JKI SM in"=w1366) -> ("error out"=w1363:errorcluster, "JKI SM out"=w1361:refnum<class "JKI SM.lvclass">)  [unwired: 6 in]
                    n489 = call "Set Visible State.vi"("error in (no error)"=w1363, "State Name"=w1360, "JKI SM in"=w1361) -> ("error out"=w1364:errorcluster, "JKI SM out"=w1365:refnum<class "JKI SM.lvclass">)  [unwired: 7 in]
                    n490 = call "Destroy.vi"("error in (no error)"=w1364, "JKI SM in"=w1365) -> ("error out"=w1362:errorcluster)  [unwired: 9 in]
                  }
                }
              }
            }
          }
          frame "EventStructure" {
            w1380 = refnum<vi> refnum  # EventStructure
            n491 = To More Specific Class(target class=w1380, reference=w1379, error in=w1377) -> (specific class reference=w1378:refnum<vi>, error out=w1376:errorcluster)
            n492 = Search 1D Array(1D array=w1383, element=w1381) -> (index of element=w1374:i32)  [unwired: 1 out]
            n493 = invoke class="EvntStruct" method="Duplicate Frame"(reference=w1378, error in=w1376, "Frame Index"=w1374) -> (reference out=w1375:refnum<vi>, error out=w1372:errorcluster)  [unwired: 1 in, 2 out]
            n494 = Increment(x=w1374) -> (x+1=w1373:i32)
            n495 = property class="EvntStruct"(reference=w1375, error in=w1372, "VisFrame"=w1373) -> (error out=w1371:errorcluster)  [unwired: 1 out]
          }
        }
        n496 = call <vilib>:"Add State(s) to Queue__jki_lib_state_machine.vi"("State(s) in Front (\"\")"=w1314, "State(s) in (\"\")"=w1316) -> ("States Out"=w1315:string)  [unwired: 13 in]
      }
      frame "Script: Find Callers" {
        n497 = Unbundle By Name(w1396) -> ("Structure Type"=w1388:T7, "FrameNames"=w1395:string[], "StructRef"=w1390:refnum<vi>)
        n498 = call "Parse State from Frame Name.vi"("Frame or State Name"=w1387) -> ("is a Category Frame?"=w1384:bool, "State Name"=w1385:string, "Category Name"=w1386:string)  [unwired: 6 in, 2 out]
        n499 = case shown="\"CaseStructure\", Default" w1388 {
          tunnel: w1395 -> [_ _]
          tunnel: [w1399 w1410] -> w1394
          tunnel: w1386 -> [_ _]
          tunnel: [_ ""] -> w1391
          tunnel: w1387 -> [w1397 _]
          tunnel: w1390 -> [w1408 w1412]
          tunnel: w1389 -> [w1407 w1411]
          tunnel: w1385 -> [_ _]
          tunnel: w1384 -> [_ _]
          frame "CaseStructure", Default {
            w1409 = refnum<vi> refnum  # CaseStructure
            n500 = To More Specific Class(target class=w1409, reference=w1408, error in=w1407) -> (specific class reference=w1406:refnum<vi>, error out=w1403:errorcluster)
            n501 = call "Create (From Structure).vi"("error in (no error)"=w1403, "Structure"=w1406) -> ("error out"=w1404:errorcluster, "JKI SM out"=w1405:refnum<class "JKI SM.lvclass">)  [unwired: 8 in]
            n502 = control-ref of="This VI"() -> (w1398:refnum<vi>)
            n503 = call "Find All Callers of State.vi"("error in (no error)"=w1404, "State Name"=w1397, "JKI SM in"=w1405) -> ("error out"=w1400:errorcluster, "Callers"=w1401:T15, "JKI SM out"=w1402:refnum<class "JKI SM.lvclass">)  [unwired: 6 in]
            n504 = call "Open Search Results Dialog.vi"("VI Refnum"=w1398, "error in (no error)"=w1400, "Callers"=w1401, "State"=w1397, "JKI SM in"=w1402) -> ("error out"=w1399:errorcluster)  [unwired: 6 in]
          }
          frame "EventStructure" {
            w1413 = refnum<vi> refnum  # EventStructure
            n505 = To More Specific Class(target class=w1413, reference=w1412, error in=w1411) -> (error out=w1410:errorcluster)  [unwired: 1 out]
          }
        }
        n506 = call <vilib>:"Add State(s) to Queue__jki_lib_state_machine.vi"("State(s) in Front (\"\")"=w1391, "State(s) in (\"\")"=w1393) -> ("States Out"=w1392:string)  [unwired: 13 in]
      }
      frame "Script: rename strings in VI" {
        # "Replace all calls to the old state name with the new one."
        n507 = Unbundle By Name(w1431) -> ("CaseStrVI Ref"=w1426:refnum<vi>)
        n508 = Match Pattern(string=w1423, regular expression=",") -> (before substring=w1417:string, after substring=w1419:string)  [unwired: 1 in, 2 out]
        n509 = Search and Replace String(replace all?=TRUE ("replace all? (F)"), input string=w1417, search string="\"") -> (result string=w1416:string)  [unwired: 5 in, 3 out]
        n510 = call <vilib>:"TRef Traverse for References.vi"("Traverse Target"=TRef_TravTarget."BD", "error in (no error)"=w1421, "Class Name"="StringConstant", "VI Refnum"=w1426) -> ("error out"=w1424:errorcluster, "References"=w1425:refnum<vi>[])  [unwired: 1 in, 5 out]
        n511 = for {
          tunnel: w1425 -> [w1451] mode=indexing
          tunnel: w1424 -> [w1448]
          tunnel: w1416 -> [w1434]
          tunnel: w1419 -> [w1433]
          tunnel: [w1436] -> w1420
          w1449 = refnum<vi> refnum  # StringConstant
          n512 = To More Specific Class(target class=w1449, reference=w1451, error in=w1448) -> (specific class reference=w1450:refnum<vi>, error out=w1447:errorcluster)
          n513 = property class="StrCnst"(reference=w1450, error in=w1447) -> (reference out=w1440:refnum<vi>, error out=w1443:errorcluster, "Value"=w1446:variant)
          n514 = Variant To Data(error in=w1443, type="", Variant=w1446) -> (data=w1435:string, error out=w1444:errorcluster)
          n515 = Search and Replace String(replace all?=TRUE ("replace all? (F)"), input string=w1435, search string=w1434, replace string=w1433, error in=w1444) -> (result string=w1432:string, error out=w1441:errorcluster)  [unwired: 3 in, 2 out]
          n516 = To Variant(anything=w1432) -> (Variant=w1439:variant)
          n517 = property class="StrCnst"(reference=w1440, error in=w1441, "Value"=w1439) -> (reference out=w1437:refnum<vi>, error out=w1438:errorcluster)
          n518 = Close Reference(reference=w1437, error in (no error)=w1438) -> (error out=w1436:errorcluster)
        }
        n519 = call <vilib>:"Add State(s) to Queue__jki_lib_state_machine.vi"("State(s) in (\"\")"=w1430) -> ("States Out"=w1429:string)  [unwired: 14 in]
      }
      frame "Script: process drag-copy" {
        # "New frame index >>"
        # "Index of original frame"
        # "Find case name"
        n520 = Unbundle By Name(w1468) -> ("FrameNames"=w1462:string[], "Cases"=w1467:refnum<vi>)
        n521 = property class="Tree (strict)"(reference=w1467, error in=w1466) -> (error out=w1460:errorcluster, "All Tags"=w1453:string[])  [unwired: 1 out]
        n522 = for {
          tunnel: w1453 -> [w1474] mode=indexing
          tunnel: w1462 -> [w1475]
          shift-right: [w1469] -> w1457
          shift-left: 0 -> [w1471]
          i -> [w1470]
          # "Find new case"
          n523 = Search 1D Array(1D array=w1475, element=w1474) -> (index of element=w1473:i32)  [unwired: 1 out]
          n524 = Greater Than 0?(x=w1473) -> (x > 0?=w1472:bool)
          n525 = Select(t=w1471, s=w1472, f=w1470) -> (s? t:f=w1469:i32)
        }
        n526 = Bundle By Name(cluster=w1468, "FrameNames"=w1453) -> (w1454:T12)
        n527 = Index Array(array=w1453, index=w1457) -> (element=w1464:string)
        n528 = Match Pattern(string=w1464, regular expression="_1") -> (before substring=w1461:string)  [unwired: 4 out]
        n529 = Search 1D Array(1D array=w1462, element=w1461) -> (index of element=w1458:i32)  [unwired: 1 out]
        n530 = Format Into String(format string="Macro: copy frame >> %d,%d", w1458, w1457) -> (resulting string=w1452:string)  [unwired: 2 in, 1 out]
        n531 = call <vilib>:"Add State(s) to Queue__jki_lib_state_machine.vi"("State(s) in Front (\"\")"=w1452, "State(s) in (\"\")"=w1456) -> ("States Out"=w1455:string)  [unwired: 1 in, 12 out]
      }
      frame "Script: copy frame" {
        n532 = Unbundle By Name(w1495) -> ("Structure Type"=w1476:T7, "SectHdr"=w1484:string, "FrameNames"=w1486:string[], "StructRef"=w1494:refnum<vi>, "Structure Type"=w1477:T7)
        n533 = Scan From String(format string="%d,%d", input string=w1493) -> (output 1=w1490:i32, output 2=w1491:i32)  [unwired: 2 in, 5 out]
        n534 = call "PromptUserWithDefault.vi"("Structure Type"=w1476, "Section"=w1484) -> ("OK"=w1485:bool, "NewTag 2"=w1481:string)  [unwired: 2 in, 6 out]
        n535 = Format Into String(format string="\"%s\"", w1481) -> (resulting string=w1480:string)  [unwired: 2 in, 1 out]
        n536 = case shown="True" w1485 {
          tunnel: w1494 -> [_ w1510]
          tunnel: w1491 -> [_ w1499]
          tunnel: w1490 -> [_ w1509]
          tunnel: w1478 -> [w1496 w1508]
          tunnel: w1486 -> [_ w1501]
          tunnel: w1481 -> [_ w1500]
          tunnel: [w1496 w1502] -> w1479
          tunnel: w1477 -> [_ w1497]
          frame False {
            # "User cancelled the operation."
          }
          frame True {
            n537 = for {
              tunnel: [w1511] -> w1503 mode=indexing
              tunnel: w1501 -> [_] mode=indexing
              i -> [w1511]
            }
            n538 = Increment(x=w1509) -> (x+1=w1506:i32)
            n539 = Delete From Array(array=w1503, index=w1506) -> (deleted portion=w1505:i32, array with subset deleted=w1507:i32[])  [unwired: 1 in]
            n540 = Insert Into Array(array=w1507, index=w1499, new element=w1505) -> (w1504:i32[])
            n541 = Replace Array Subset(array=w1501, new element=w1500, index=w1499) -> (w1498:string[])
            n542 = call "Script - copy frame.vi"("FrameNames"=w1498, "Array"=w1504, "error in"=w1508, "Structure Type"=w1497, "Numeric"=w1509, "StructRef"=w1510) -> ("error out"=w1502:errorcluster)  [unwired: 5 in]
          }
        }
        n543 = Bundle By Name(cluster=w1495, "tag"=w1480) -> (w1483:T12)
        n544 = call <vilib>:"Add State(s) to Queue__jki_lib_state_machine.vi"("State(s) in Front (\"\")"="Macro: update list\nMacro: update list" ("State(s) in Front (\"\")"), "State(s) in (\"\")"=w1489) -> ("States Out"=w1488:string)  [unwired: 1 in, 12 out]
      }
      frame "Script: drop state name" {
      }
      frame "Script: end undo" {
        n545 = Unbundle By Name(w1520) -> ("CaseStrVI Ref"=w1518:refnum<vi>)
        n546 = Bundle By Name(cluster=w1520, "Undo Transaction"=FALSE) -> (w1516:T12)
        n547 = invoke class="VI" method="Transaction.End Undo"(reference=w1518, error in=w1519) -> (error out=w1522:errorcluster)  [unwired: 1 in, 2 out]
        n548 = call <vilib>:"Clear Errors.vi"("error in (no error)"=w1522) -> ("error out"=w1517:errorcluster)  [unwired: 6 in]
      }
      frame "Script: do undo" {
        n549 = Unbundle By Name(w1526) -> ("CaseStrVI Ref"=w1524:refnum<vi>)
        n550 = invoke class="VI" method="Transaction.Undo"(reference=w1524, error in=w1525) -> (error out=w1528:errorcluster)  [unwired: 1 in, 2 out]
        n551 = call <vilib>:"Clear Errors.vi"("error in (no error)"=w1528) -> ("error out"=w1523:errorcluster)  [unwired: 6 in]
      }
      frame "Script: fail undo" {
        n552 = Unbundle By Name(w1534) -> ("CaseStrVI Ref"=w1532:refnum<vi>)
        n553 = Bundle By Name(cluster=w1534, "Undo Transaction"=FALSE) -> (w1530:T12)
        n554 = invoke class="VI" method="Transaction.Fail"(reference=w1532, error in=w1533) -> (error out=w1536:errorcluster)  [unwired: 1 in, 2 out]
        n555 = call <vilib>:"Clear Errors.vi"("error in (no error)"=w1536) -> ("error out"=w1531:errorcluster)  [unwired: 6 in]
      }
      frame "Script: append string" {
        w1540 = refnum<vi> refnum  # CaseStructure
        n556 = Unbundle By Name(w1560) -> ("StructRef"=w1539:refnum<vi>, "tag"=w1546:string, "CaseStrVI Ref"=w1558:refnum<vi>)
        n557 = property class="VI"(reference=w1558, error in=w1559) -> (error out=w1555:errorcluster, "Diagram"=w1557:refnum<vi>)  [unwired: 1 out]
        n558 = property class="TopLvlDiag"(reference=w1557, error in=w1555) -> (error out=w1552:errorcluster, "SelList[]"=w1556:refnum<vi>[])  [unwired: 1 out]
        n559 = Search and Replace String(replace all?=TRUE ("replace all? (F)"), input string=w1546, search string="\"") -> (result string=w1547:string)  [unwired: 5 in, 3 out]
        n560 = To More Specific Class(target class=w1540, reference=w1539) -> (specific class reference=w1538:refnum<vi>, error out=w1537:errorcluster)  [unwired: 1 in]
        n561 = call "JKI Arguments Used.vi"("error in"=w1537, "CaseSel Refnum"=w1538) -> ("error out"=w1542:errorcluster, "Arguments used?"=w1543:bool)  [unwired: 8 in]
        n562 = call "RCF Case Select"("Enable"=w1543, "error in (no error)"=w1542) -> ("Argument"=w1541:string)  [unwired: 15 in, 2 out]
        n563 = Array Size(array=w1556) -> (size(s)=w1554:i32)
        n564 = Index Array(array=w1556) -> (element=w1551:refnum<vi>)  [unwired: 1 in]
        n565 = case shown="1" w1554 {
          tunnel: [w1561 w1565] -> w1553
          tunnel: w1552 -> [w1561 w1569]
          tunnel: w1551 -> [_ w1568]
          tunnel: w1547 -> [_ w1563]
          tunnel: w1541 -> [_ w1562]
          frame 0, Default {
          }
          frame 1 {
            w1567 = refnum<vi> refnum  # StringConstant
            n566 = To More Specific Class(target class=w1567, reference=w1568, error in=w1569) -> (specific class reference=w1566:refnum<vi>, error out=w1564:errorcluster)
            n567 = case shown="No Error" w1564 {
              selector: w1564 -> [w1583 w1591]
              tunnel: w1566 -> [w1589 _]
              tunnel: [w1584 w1590] -> w1565
              tunnel: w1563 -> [w1580 _]
              tunnel: w1562 -> [w1572 _]
              frame No Error {
                n568 = property class="StrCnst"(reference=w1589, error in=w1583) -> (reference out=w1585:refnum<vi>, error out=w1588:errorcluster, "Value"=w1579:variant)
                n569 = Empty String/Path?(string/path=w1572) -> (empty?=w1575:bool)
                n570 = Format Into String(format string=" >> %s", w1572) -> (resulting string=w1571:string)  [unwired: 2 in, 1 out]
                n571 = Select(t="", s=w1575, f=w1571) -> (s? t:f=w1570:string)
                n572 = Variant To Data(error in=w1588, type="", Variant=w1579) -> (data=w1581:string, error out=w1586:errorcluster)
                n573 = Format Into String(format string="%s\n%s%s", w1581, w1580, w1570) -> (resulting string=w1577:string)  [unwired: 2 in, 1 out]
                n574 = call <vilib>:"Trim Whitespace.vi"("string"=w1577) -> ("trimmed string"=w1576:string)  [unwired: 1 in]
                n575 = To Variant(anything=w1576) -> (Variant=w1578:variant)
                n576 = property class="StrCnst"(reference=w1585, error in=w1586, "Value"=w1578) -> (error out=w1584:errorcluster)  [unwired: 1 out]
              }
              frame Error {
                # "I don't care..."
                n577 = call <vilib>:"Clear Errors.vi"("error in (no error)"=w1591) -> ("error out"=w1590:errorcluster)  [unwired: 6 in]
              }
            }
          }
        }
        n578 = call <vilib>:"Add State(s) to Queue__jki_lib_state_machine.vi"("State(s) in Front (\"\")"="Script: highlight" ("State(s) in Front (\"\")"), "State(s) in (\"\")"=w1550) -> ("States Out"=w1549:string)  [unwired: 13 in]
      }
      frame "Script: highlight" {
        n579 = Unbundle By Name(w1599) -> ("CaseStrVI Ref"=w1595:refnum<vi>)
        n580 = property class="VI"(reference=w1595, error in=w1596) -> (error out=w1597:errorcluster, "Diagram"=w1598:refnum<vi>)  [unwired: 1 out]
        n581 = property class="TopLvlDiag"(reference=w1598, error in=w1597) -> (error out=w1593:errorcluster, "SelList[]"=w1592:refnum<vi>[])  [unwired: 1 out]
        n582 = for {
          tunnel: [w1601] -> w1594
          tunnel: w1593 -> [w1603]
          tunnel: w1592 -> [w1602] mode=indexing
          n583 = invoke class="GObj" method="ObjHighlight"(reference=w1602, error in=w1603) -> (error out=w1601:errorcluster)  [unwired: 1 in, 2 out]
        }
      }
    }
  }
  n584 = call <vilib>:"Simple Error Handler.vi"("error in (no error)"=w3) -> ()  [unwired: 4 in, 5 out]
